vi "LCS kNN.vi"() -> ()   [LabVIEW 2014]
uses:
  <vilib>/Utility/file.llb/Write To Spreadsheet File (string).vi
panel:
  in  "4 groups":string[][](array[string])=[["0 1 0 1 0 3 0", "10", "1"], ["0 -1 1 0 1 0 3 0", "10", "1"], ["0 1 -1 0 1 0 3 0", "10", "1"], ["0 -4 1 0 1 0 3 0", "10", "1"], ["0 1 -4 0 1 0 3 0", "10", "1"], ["0 1 0 -1 1 0 3 0", "10", "1"], ["0 -1 1 0 -1 1 0 3 0", "10", "1"], ["0 1 -1 0 -1 1 0 3 0", "10", "1"], ["0 -4 1 0 -1 1 0 3 0", "10", "1"], ["0 1 -4 0 -1 1 0 3 0", "10", "1"], ["0 1 0 1 -1 0 3 0", "10", "1"], ["0 -1 1 0 1 -1 0 3 0", "10", "1"], ["0 1 -1 0 1 -1 0 3 0", "10", "1"], ["0 -4 1 0 1 -1 0 3 0", "10", "1"], ["0 1 -4 0 1 -1 0 3 0", "10", "1"], ["0 1 0 -4 1 0 3 0", "10", "1"], ["0 -1 1 0 -4 1 0 3 0", "10", "1"], ["0 1 -1 0 -4 1 0 3 0", "10", "1"], ["0 -4 1 0 -4 1 0 3 0", "10", "1"], ["0 1 -4 0 -4 1 0 3 0", "10", "1"], ["0 1 0 1 -4 0 3 0", "10", "1"], ["0 -1 1 0 1 -4 0 3 0", "10", "1"], ["0 1 -1 0 1 -4 0 3 0", "10", "1"], ["0 -4 1 0 1 -4 0 3 0", "10", "1"], ["0 1 -4 0 1 -4 0 3 0", "10", "1"], ["0 1 0 1 0 -2 3 0", "10", "1"], ["0 -1 1 0 1 0 -2 3 0", "10", "1"], ["0 1 -1 0 1 0 -2 3 0", "10", "1"], ["0 -4 1 0 1 0 -2 3 0", "10", "1"], ["0 1 -4 0 1 0 -2 3 0", "10", "1"], ["0 1 0 -1 1 0 -2 3 0", "10", "1"], ["0 -1 1 0 -1 1 0 -2 3 0", "10", "1"], ["0 1 -1 0 -1 1 0 -2 3 0", "10", "1"], ["0 -4 1 0 -1 1 0 -2 3 0", "10", "1"], ["0 1 -4 0 -1 1 0 -2 3 0", "10", "1"], ["0 1 0 1 -1 0 -2 3 0", "10", "1"], ["0 -1 1 0 1 -1 0 -2 3 0", "10", "1"], ["0 1 -1 0 1 -1 0 -2 3 0", "10", "1"], ["0 -4 1 0 1 -1 0 -2 3 0", "10", "1"], ["0 1 -4 0 1 -1 0 -2 3 0", "10", "1"], ["0 1 0 -4 1 0 -2 3 0", "10", "1"], ["0 -1 1 0 -4 1 0 -2 3 0", "10", "1"], ["0 1 -1 0 -4 1 0 -2 3 0", "10", "1"], ["0 -4 1 0 -4 1 0 -2 3 0", "10", "1"], ["0 1 -4 0 -4 1 0 -2 3 0", "10", "1"], ["0 1 0 1 -4 0 -2 3 0", "10", "1"], ["0 -1 1 0 1 -4 0 -2 3 0", "10", "1"], ["0 1 -1 0 1 -4 0 -2 3 0", "10", "1"], ["0 -4 1 0 1 -4 0 -2 3 0", "10", "1"], ["0 1 -4 0 1 -4 0 -2 3 0", "10", "1"], ["0 1 0 1 0 3 -2 0", "10", "1"], ["0 -1 1 0 1 0 3 -2 0", "10", "1"], ["0 1 -1 0 1 0 3 -2 0", "10", "1"], ["0 -4 1 0 1 0 3 -2 0", "10", "1"], ["0 1 -4 0 1 0 3 -2 0", "10", "1"], ["0 1 0 -1 1 0 3 -2 0", "10", "1"], ["0 -1 1 0 -1 1 0 3 -2 0", "10", "1"], ["0 1 -1 0 -1 1 0 3 -2 0", "10", "1"], ["0 -4 1 0 -1 1 0 3 -2 0", "10", "1"], ["0 1 -4 0 -1 1 0 3 -2 0", "10", "1"], ["0 1 0 1 -1 0 3 -2 0", "10", "1"], ["0 -1 1 0 1 -1 0 3 -2 0", "10", "1"], ["0 1 -1 0 1 -1 0 3 -2 0", "10", "1"], ["0 -4 1 0 1 -1 0 3 -2 0", "10", "1"], ["0 1 -4 0 1 -1 0 3 -2 0", "10", "1"], ["0 1 0 -4 1 0 3 -2 0", "10", "1"], ["0 -1 1 0 -4 1 0 3 -2 0", "10", "1"], ["0 1 -1 0 -4 1 0 3 -2 0", "10", "1"], ["0 -4 1 0 -4 1 0 3 -2 0", "10", "1"], ["0 1 -4 0 -4 1 0 3 -2 0", "10", "1"], ["0 1 0 1 -4 0 3 -2 0", "10", "1"], ["0 -1 1 0 1 -4 0 3 -2 0", "10", "1"], ["0 1 -1 0 1 -4 0 3 -2 0", "10", "1"], ["0 -4 1 0 1 -4 0 3 -2 0", "10", "1"], ["0 1 -4 0 1 -4 0 3 -2 0", "10", "1"], ["0 1 0 1 0 -3 3 0", "10", "1"], ["0 -1 1 0 1 0 -3 3 0", "10", "1"], ["0 1 -1 0 1 0 -3 3 0", "10", "1"], ["0 -4 1 0 1 0 -3 3 0", "10", "1"], ["0 1 -4 0 1 0 -3 3 0", "10", "1"], ["0 1 0 -1 1 0 -3 3 0", "10", "1"], ["0 -1 1 0 -1 1 0 -3 3 0", "10", "1"], ["0 1 -1 0 -1 1 0 -3 3 0", "10", "1"], ["0 -4 1 0 -1 1 0 -3 3 0", "10", "1"], ["0 1 -4 0 -1 1 0 -3 3 0", "10", "1"], ["0 1 0 1 -1 0 -3 3 0", "10", "1"], ["0 -1 1 0 1 -1 0 -3 3 0", "10", "1"], ["0 1 -1 0 1 -1 0 -3 3 0", "10", "1"], ["0 -4 1 0 1 -1 0 -3 3 0", "10", "1"], ["0 1 -4 0 1 -1 0 -3 3 0", "10", "1"], ["0 1 0 -4 1 0 -3 3 0", "10", "1"], ["0 -1 1 0 -4 1 0 -3 3 0", "10", "1"], ["0 1 -1 0 -4 1 0 -3 3 0", "10", "1"], ["0 -4 1 0 -4 1 0 -3 3 0", "10", "1"], ["0 1 -4 0 -4 1 0 -3 3 0", "10", "1"], ["0 1 0 1 -4 0 -3 3 0", "10", "1"], ["0 -1 1 0 1 -4 0 -3 3 0", "10", "1"], ["0 1 -1 0 1 -4 0 -3 3 0", "10", "1"], ["0 -4 1 0 1 -4 0 -3 3 0", "10", "1"], ["0 1 -4 0 1 -4 0 -3 3 0", "10", "1"], ["0 1 0 1 0 3 -3 0", "10", "1"], ["0 -1 1 0 1 0 3 -3 0", "10", "1"], ["0 1 -1 0 1 0 3 -3 0", "10", "1"], ["0 -4 1 0 1 0 3 -3 0", "10", "1"], ["0 1 -4 0 1 0 3 -3 0", "10", "1"], ["0 1 0 -1 1 0 3 -3 0", "10", "1"], ["0 -1 1 0 -1 1 0 3 -3 0", "10", "1"], ["0 1 -1 0 -1 1 0 3 -3 0", "10", "1"], ["0 -4 1 0 -1 1 0 3 -3 0", "10", "1"], ["0 1 -4 0 -1 1 0 3 -3 0", "10", "1"], ["0 1 0 1 -1 0 3 -3 0", "10", "1"], ["0 -1 1 0 1 -1 0 3 -3 0", "10", "1"], ["0 1 -1 0 1 -1 0 3 -3 0", "10", "1"], ["0 -4 1 0 1 -1 0 3 -3 0", "10", "1"], ["0 1 -4 0 1 -1 0 3 -3 0", "10", "1"], ["0 1 0 -4 1 0 3 -3 0", "10", "1"], ["0 -1 1 0 -4 1 0 3 -3 0", "10", "1"], ["0 1 -1 0 -4 1 0 3 -3 0", "10", "1"], ["0 -4 1 0 -4 1 0 3 -3 0", "10", "1"], ["0 1 -4 0 -4 1 0 3 -3 0", "10", "1"], ["0 1 0 1 -4 0 3 -3 0", "10", "1"], ["0 -1 1 0 1 -4 0 3 -3 0", "10", "1"], ["0 1 -1 0 1 -4 0 3 -3 0", "10", "1"], ["0 -4 1 0 1 -4 0 3 -3 0", "10", "1"], ["0 1 -4 0 1 -4 0 3 -3 0", "10", "1"], ["0 1 0 3 0 1 0", "10", "2"], ["0 -1 1 0 3 0 1 0", "10", "2"], ["0 1 -1 0 3 0 1 0", "10", "2"], ["0 -4 1 0 3 0 1 0", "10", "2"], ["0 1 -4 0 3 0 1 0", "10", "2"], ["0 1 0 -2 3 0 1 0", "10", "2"], ["0 -1 1 0 -2 3 0 1 0", "10", "2"], ["0 1 -1 0 -2 3 0 1 0", "10", "2"], ["0 -4 1 0 -2 3 0 1 0", "10", "2"], ["0 1 -4 0 -2 3 0 1 0", "10", "2"], ["0 1 0 3 -2 0 1 0", "10", "2"], ["0 -1 1 0 3 -2 0 1 0", "10", "2"], ["0 1 -1 0 3 -2 0 1 0", "10", "2"], ["0 -4 1 0 3 -2 0 1 0", "10", "2"], ["0 1 -4 0 3 -2 0 1 0", "10", "2"], ["0 1 0 -3 3 0 1 0", "10", "2"], ["0 -1 1 0 -3 3 0 1 0", "10", "2"], ["0 1 -1 0 -3 3 0 1 0", "10", "2"], ["0 -4 1 0 -3 3 0 1 0", "10", "2"], ["0 1 -4 0 -3 3 0 1 0", "10", "2"], ["0 1 0 3 -3 0 1 0", "10", "2"], ["0 -1 1 0 3 -3 0 1 0", "10", "2"], ["0 1 -1 0 3 -3 0 1 0", "10", "2"], ["0 -4 1 0 3 -3 0 1 0", "10", "2"], ["0 1 -4 0 3 -3 0 1 0", "10", "2"], ["0 1 0 3 0 -1 1 0", "10", "2"], ["0 -1 1 0 3 0 -1 1 0", "10", "2"], ["0 1 -1 0 3 0 -1 1 0", "10", "2"], ["0 -4 1 0 3 0 -1 1 0", "10", "2"], ["0 1 -4 0 3 0 -1 1 0", "10", "2"], ["0 1 0 -2 3 0 -1 1 0", "10", "2"], ["0 -1 1 0 -2 3 0 -1 1 0", "10", "2"], ["0 1 -1 0 -2 3 0 -1 1 0", "10", "2"], ["0 -4 1 0 -2 3 0 -1 1 0", "10", "2"], ["0 1 -4 0 -2 3 0 -1 1 0", "10", "2"], ["0 1 0 3 -2 0 -1 1 0", "10", "2"], ["0 -1 1 0 3 -2 0 -1 1 0", "10", "2"], ["0 1 -1 0 3 -2 0 -1 1 0", "10", "2"], ["0 -4 1 0 3 -2 0 -1 1 0", "10", "2"], ["0 1 -4 0 3 -2 0 -1 1 0", "10", "2"], ["0 1 0 -3 3 0 -1 1 0", "10", "2"], ["0 -1 1 0 -3 3 0 -1 1 0", "10", "2"], ["0 1 -1 0 -3 3 0 -1 1 0", "10", "2"], ["0 -4 1 0 -3 3 0 -1 1 0", "10", "2"], ["0 1 -4 0 -3 3 0 -1 1 0", "10", "2"], ["0 1 0 3 -3 0 -1 1 0", "10", "2"], ["0 -1 1 0 3 -3 0 -1 1 0", "10", "2"], ["0 1 -1 0 3 -3 0 -1 1 0", "10", "2"], ["0 -4 1 0 3 -3 0 -1 1 0", "10", "2"], ["0 1 -4 0 3 -3 0 -1 1 0", "10", "2"], ["0 1 0 3 0 1 -1 0", "10", "2"], ["0 -1 1 0 3 0 1 -1 0", "10", "2"], ["0 1 -1 0 3 0 1 -1 0", "10", "2"], ["0 -4 1 0 3 0 1 -1 0", "10", "2"], ["0 1 -4 0 3 0 1 -1 0", "10", "2"], ["0 1 0 -2 3 0 1 -1 0", "10", "2"], ["0 -1 1 0 -2 3 0 1 -1 0", "10", "2"], ["0 1 -1 0 -2 3 0 1 -1 0", "10", "2"], ["0 -4 1 0 -2 3 0 1 -1 0", "10", "2"], ["0 1 -4 0 -2 3 0 1 -1 0", "10", "2"], ["0 1 0 3 -2 0 1 -1 0", "10", "2"], ["0 -1 1 0 3 -2 0 1 -1 0", "10", "2"], ["0 1 -1 0 3 -2 0 1 -1 0", "10", "2"], ["0 -4 1 0 3 -2 0 1 -1 0", "10", "2"], ["0 1 -4 0 3 -2 0 1 -1 0", "10", "2"], ["0 1 0 -3 3 0 1 -1 0", "10", "2"], ["0 -1 1 0 -3 3 0 1 -1 0", "10", "2"], ["0 1 -1 0 -3 3 0 1 -1 0", "10", "2"], ["0 -4 1 0 -3 3 0 1 -1 0", "10", "2"], ["0 1 -4 0 -3 3 0 1 -1 0", "10", "2"], ["0 1 0 3 -3 0 1 -1 0", "10", "2"], ["0 -1 1 0 3 -3 0 1 -1 0", "10", "2"], ["0 1 -1 0 3 -3 0 1 -1 0", "10", "2"], ["0 -4 1 0 3 -3 0 1 -1 0", "10", "2"], ["0 1 -4 0 3 -3 0 1 -1 0", "10", "2"], ["0 1 0 3 0 -4 1 0", "10", "2"], ["0 -1 1 0 3 0 -4 1 0", "10", "2"], ["0 1 -1 0 3 0 -4 1 0", "10", "2"], ["0 -4 1 0 3 0 -4 1 0", "10", "2"], ["0 1 -4 0 3 0 -4 1 0", "10", "2"], ["0 1 0 -2 3 0 -4 1 0", "10", "2"], ["0 -1 1 0 -2 3 0 -4 1 0", "10", "2"], ["0 1 -1 0 -2 3 0 -4 1 0", "10", "2"], ["0 -4 1 0 -2 3 0 -4 1 0", "10", "2"], ["0 1 -4 0 -2 3 0 -4 1 0", "10", "2"], ["0 1 0 3 -2 0 -4 1 0", "10", "2"], ["0 -1 1 0 3 -2 0 -4 1 0", "10", "2"], ["0 1 -1 0 3 -2 0 -4 1 0", "10", "2"], ["0 -4 1 0 3 -2 0 -4 1 0", "10", "2"], ["0 1 -4 0 3 -2 0 -4 1 0", "10", "2"], ["0 1 0 -3 3 0 -4 1 0", "10", "2"], ["0 -1 1 0 -3 3 0 -4 1 0", "10", "2"], ["0 1 -1 0 -3 3 0 -4 1 0", "10", "2"], ["0 -4 1 0 -3 3 0 -4 1 0", "10", "2"], ["0 1 -4 0 -3 3 0 -4 1 0", "10", "2"], ["0 1 0 3 -3 0 -4 1 0", "10", "2"], ["0 -1 1 0 3 -3 0 -4 1 0", "10", "2"], ["0 1 -1 0 3 -3 0 -4 1 0", "10", "2"], ["0 -4 1 0 3 -3 0 -4 1 0", "10", "2"], ["0 1 -4 0 3 -3 0 -4 1 0", "10", "2"], ["0 1 0 3 0 1 -4 0", "10", "2"], ["0 -1 1 0 3 0 1 -4 0", "10", "2"], ["0 1 -1 0 3 0 1 -4 0", "10", "2"], ["0 -4 1 0 3 0 1 -4 0", "10", "2"], ["0 1 -4 0 3 0 1 -4 0", "10", "2"], ["0 1 0 -2 3 0 1 -4 0", "10", "2"], ["0 -1 1 0 -2 3 0 1 -4 0", "10", "2"], ["0 1 -1 0 -2 3 0 1 -4 0", "10", "2"], ["0 -4 1 0 -2 3 0 1 -4 0", "10", "2"], ["0 1 -4 0 -2 3 0 1 -4 0", "10", "2"], ["0 1 0 3 -2 0 1 -4 0", "10", "2"], ["0 -1 1 0 3 -2 0 1 -4 0", "10", "2"], ["0 1 -1 0 3 -2 0 1 -4 0", "10", "2"], ["0 -4 1 0 3 -2 0 1 -4 0", "10", "2"], ["0 1 -4 0 3 -2 0 1 -4 0", "10", "2"], ["0 1 0 -3 3 0 1 -4 0", "10", "2"], ["0 -1 1 0 -3 3 0 1 -4 0", "10", "2"], ["0 1 -1 0 -3 3 0 1 -4 0", "10", "2"], ["0 -4 1 0 -3 3 0 1 -4 0", "10", "2"], ["0 1 -4 0 -3 3 0 1 -4 0", "10", "2"], ["0 1 0 3 -3 0 1 -4 0", "10", "2"], ["0 -1 1 0 3 -3 0 1 -4 0", "10", "2"], ["0 1 -1 0 3 -3 0 1 -4 0", "10", "2"], ["0 -4 1 0 3 -3 0 1 -4 0", "10", "2"], ["0 1 -4 0 3 -3 0 1 -4 0", "10", "2"], ["0 3 0 3 0 1 0", "10", "3"], ["0 -2 3 0 3 0 1 0", "10", "3"], ["0 3 -2 0 3 0 1 0", "10", "3"], ["0 -3 3 0 3 0 1 0", "10", "3"], ["0 3-3 0 3 0 1 0", "10", "3"], ["0 3 0 -2 3 0 1 0", "10", "3"], ["0 -2 3 0 -2 3 0 1 0", "10", "3"], ["0 3 -2 0 -2 3 0 1 0", "10", "3"], ["0 -3 3 0 -2 3 0 1 0", "10", "3"], ["0 3-3 0 -2 3 0 1 0", "10", "3"], ["0 3 0 3 -2 0 1 0", "10", "3"], ["0 -2 3 0 3 -2 0 1 0", "10", "3"], ["0 3 -2 0 3 -2 0 1 0", "10", "3"], ["0 -3 3 0 3 -2 0 1 0", "10", "3"], ["0 3-3 0 3 -2 0 1 0", "10", "3"], ["0 3 0 -3 3 0 1 0", "10", "3"], ["0 -2 3 0 -3 3 0 1 0", "10", "3"], ["0 3 -2 0 -3 3 0 1 0", "10", "3"], ["0 -3 3 0 -3 3 0 1 0", "10", "3"], ["0 3-3 0 -3 3 0 1 0", "10", "3"], ["0 3 0 3 -3 0 1 0", "10", "3"], ["0 -2 3 0 3 -3 0 1 0", "10", "3"], ["0 3 -2 0 3 -3 0 1 0", "10", "3"], ["0 -3 3 0 3 -3 0 1 0", "10", "3"], ["0 3-3 0 3 -3 0 1 0", "10", "3"], ["0 3 0 3 0 -1 1 0", "10", "3"], ["0 -2 3 0 3 0 -1 1 0", "10", "3"], ["0 3 -2 0 3 0 -1 1 0", "10", "3"], ["0 -3 3 0 3 0 -1 1 0", "10", "3"], ["0 3-3 0 3 0 -1 1 0", "10", "3"], ["0 3 0 -2 3 0 -1 1 0", "10", "3"], ["0 -2 3 0 -2 3 0 -1 1 0", "10", "3"], ["0 3 -2 0 -2 3 0 -1 1 0", "10", "3"], ["0 -3 3 0 -2 3 0 -1 1 0", "10", "3"], ["0 3-3 0 -2 3 0 -1 1 0", "10", "3"], ["0 3 0 3 -2 0 -1 1 0", "10", "3"], ["0 -2 3 0 3 -2 0 -1 1 0", "10", "3"], ["0 3 -2 0 3 -2 0 -1 1 0", "10", "3"], ["0 -3 3 0 3 -2 0 -1 1 0", "10", "3"], ["0 3-3 0 3 -2 0 -1 1 0", "10", "3"], ["0 3 0 -3 3 0 -1 1 0", "10", "3"], ["0 -2 3 0 -3 3 0 -1 1 0", "10", "3"], ["0 3 -2 0 -3 3 0 -1 1 0", "10", "3"], ["0 -3 3 0 -3 3 0 -1 1 0", "10", "3"], ["0 3-3 0 -3 3 0 -1 1 0", "10", "3"], ["0 3 0 3 -3 0 -1 1 0", "10", "3"], ["0 -2 3 0 3 -3 0 -1 1 0", "10", "3"], ["0 3 -2 0 3 -3 0 -1 1 0", "10", "3"], ["0 -3 3 0 3 -3 0 -1 1 0", "10", "3"], ["0 3-3 0 3 -3 0 -1 1 0", "10", "3"], ["0 3 0 3 0 1 -1 0", "10", "3"], ["0 -2 3 0 3 0 1 -1 0", "10", "3"], ["0 3 -2 0 3 0 1 -1 0", "10", "3"], ["0 -3 3 0 3 0 1 -1 0", "10", "3"], ["0 3-3 0 3 0 1 -1 0", "10", "3"], ["0 3 0 -2 3 0 1 -1 0", "10", "3"], ["0 -2 3 0 -2 3 0 1 -1 0", "10", "3"], ["0 3 -2 0 -2 3 0 1 -1 0", "10", "3"], ["0 -3 3 0 -2 3 0 1 -1 0", "10", "3"], ["0 3-3 0 -2 3 0 1 -1 0", "10", "3"], ["0 3 0 3 -2 0 1 -1 0", "10", "3"], ["0 -2 3 0 3 -2 0 1 -1 0", "10", "3"], ["0 3 -2 0 3 -2 0 1 -1 0", "10", "3"], ["0 -3 3 0 3 -2 0 1 -1 0", "10", "3"], ["0 3-3 0 3 -2 0 1 -1 0", "10", "3"], ["0 3 0 -3 3 0 1 -1 0", "10", "3"], ["0 -2 3 0 -3 3 0 1 -1 0", "10", "3"], ["0 3 -2 0 -3 3 0 1 -1 0", "10", "3"], ["0 -3 3 0 -3 3 0 1 -1 0", "10", "3"], ["0 3-3 0 -3 3 0 1 -1 0", "10", "3"], ["0 3 0 3 -3 0 1 -1 0", "10", "3"], ["0 -2 3 0 3 -3 0 1 -1 0", "10", "3"], ["0 3 -2 0 3 -3 0 1 -1 0", "10", "3"], ["0 -3 3 0 3 -3 0 1 -1 0", "10", "3"], ["0 3-3 0 3 -3 0 1 -1 0", "10", "3"], ["0 3 0 3 0 -4 1 0", "10", "3"], ["0 -2 3 0 3 0 -4 1 0", "10", "3"], ["0 3 -2 0 3 0 -4 1 0", "10", "3"], ["0 -3 3 0 3 0 -4 1 0", "10", "3"], ["0 3-3 0 3 0 -4 1 0", "10", "3"], ["0 3 0 -2 3 0 -4 1 0", "10", "3"], ["0 -2 3 0 -2 3 0 -4 1 0", "10", "3"], ["0 3 -2 0 -2 3 0 -4 1 0", "10", "3"], ["0 -3 3 0 -2 3 0 -4 1 0", "10", "3"], ["0 3-3 0 -2 3 0 -4 1 0", "10", "3"], ["0 3 0 3 -2 0 -4 1 0", "10", "3"], ["0 -2 3 0 3 -2 0 -4 1 0", "10", "3"], ["0 3 -2 0 3 -2 0 -4 1 0", "10", "3"], ["0 -3 3 0 3 -2 0 -4 1 0", "10", "3"], ["0 3-3 0 3 -2 0 -4 1 0", "10", "3"], ["0 3 0 -3 3 0 -4 1 0", "10", "3"], ["0 -2 3 0 -3 3 0 -4 1 0", "10", "3"], ["0 3 -2 0 -3 3 0 -4 1 0", "10", "3"], ["0 -3 3 0 -3 3 0 -4 1 0", "10", "3"], ["0 3-3 0 -3 3 0 -4 1 0", "10", "3"], ["0 3 0 3 -3 0 -4 1 0", "10", "3"], ["0 -2 3 0 3 -3 0 -4 1 0", "10", "3"], ["0 3 -2 0 3 -3 0 -4 1 0", "10", "3"], ["0 -3 3 0 3 -3 0 -4 1 0", "10", "3"], ["0 3-3 0 3 -3 0 -4 1 0", "10", "3"], ["0 3 0 3 0 1 -4 0", "10", "3"], ["0 -2 3 0 3 0 1 -4 0", "10", "3"], ["0 3 -2 0 3 0 1 -4 0", "10", "3"], ["0 -3 3 0 3 0 1 -4 0", "10", "3"], ["0 3-3 0 3 0 1 -4 0", "10", "3"], ["0 3 0 -2 3 0 1 -4 0", "10", "3"], ["0 -2 3 0 -2 3 0 1 -4 0", "10", "3"], ["0 3 -2 0 -2 3 0 1 -4 0", "10", "3"], ["0 -3 3 0 -2 3 0 1 -4 0", "10", "3"], ["0 3-3 0 -2 3 0 1 -4 0", "10", "3"], ["0 3 0 3 -2 0 1 -4 0", "10", "3"], ["0 -2 3 0 3 -2 0 1 -4 0", "10", "3"], ["0 3 -2 0 3 -2 0 1 -4 0", "10", "3"], ["0 -3 3 0 3 -2 0 1 -4 0", "10", "3"], ["0 3-3 0 3 -2 0 1 -4 0", "10", "3"], ["0 3 0 -3 3 0 1 -4 0", "10", "3"], ["0 -2 3 0 -3 3 0 1 -4 0", "10", "3"], ["0 3 -2 0 -3 3 0 1 -4 0", "10", "3"], ["0 -3 3 0 -3 3 0 1 -4 0", "10", "3"], ["0 3-3 0 -3 3 0 1 -4 0", "10", "3"], ["0 3 0 3 -3 0 1 -4 0", "10", "3"], ["0 -2 3 0 3 -3 0 1 -4 0", "10", "3"], ["0 3 -2 0 3 -3 0 1 -4 0", "10", "3"], ["0 -3 3 0 3 -3 0 1 -4 0", "10", "3"], ["0 3-3 0 3 -3 0 1 -4 0", "10", "3"], ["0 3 0 1 0 3 0", "10", "4"], ["0 -2 3 0 1 0 3 0", "10", "4"], ["0 3 -2 0 1 0 3 0", "10", "4"], ["0 -3 3 0 1 0 3 0", "10", "4"], ["0 3-3 0 1 0 3 0", "10", "4"], ["0 3 0 -1 1 0 3 0", "10", "4"], ["0 -2 3 0 -1 1 0 3 0", "10", "4"], ["0 3 -2 0 -1 1 0 3 0", "10", "4"], ["0 -3 3 0 -1 1 0 3 0", "10", "4"], ["0 3-3 0 -1 1 0 3 0", "10", "4"], ["0 3 0 1 -1 0 3 0", "10", "4"], ["0 -2 3 0 1 -1 0 3 0", "10", "4"], ["0 3 -2 0 1 -1 0 3 0", "10", "4"], ["0 -3 3 0 1 -1 0 3 0", "10", "4"], ["0 3-3 0 1 -1 0 3 0", "10", "4"], ["0 3 0 -4 1 0 3 0", "10", "4"], ["0 -2 3 0 -4 1 0 3 0", "10", "4"], ["0 3 -2 0 -4 1 0 3 0", "10", "4"], ["0 -3 3 0 -4 1 0 3 0", "10", "4"], ["0 3-3 0 -4 1 0 3 0", "10", "4"], ["0 3 0 1 -4 0 3 0", "10", "4"], ["0 -2 3 0 1 -4 0 3 0", "10", "4"], ["0 3 -2 0 1 -4 0 3 0", "10", "4"], ["0 -3 3 0 1 -4 0 3 0", "10", "4"], ["0 3-3 0 1 -4 0 3 0", "10", "4"], ["0 3 0 1 0 -2 3 0", "10", "4"], ["0 -2 3 0 1 0 -2 3 0", "10", "4"], ["0 3 -2 0 1 0 -2 3 0", "10", "4"], ["0 -3 3 0 1 0 -2 3 0", "10", "4"], ["0 3-3 0 1 0 -2 3 0", "10", "4"], ["0 3 0 -1 1 0 -2 3 0", "10", "4"], ["0 -2 3 0 -1 1 0 -2 3 0", "10", "4"], ["0 3 -2 0 -1 1 0 -2 3 0", "10", "4"], ["0 -3 3 0 -1 1 0 -2 3 0", "10", "4"], ["0 3-3 0 -1 1 0 -2 3 0", "10", "4"], ["0 3 0 1 -1 0 -2 3 0", "10", "4"], ["0 -2 3 0 1 -1 0 -2 3 0", "10", "4"], ["0 3 -2 0 1 -1 0 -2 3 0", "10", "4"], ["0 -3 3 0 1 -1 0 -2 3 0", "10", "4"], ["0 3-3 0 1 -1 0 -2 3 0", "10", "4"], ["0 3 0 -4 1 0 -2 3 0", "10", "4"], ["0 -2 3 0 -4 1 0 -2 3 0", "10", "4"], ["0 3 -2 0 -4 1 0 -2 3 0", "10", "4"], ["0 -3 3 0 -4 1 0 -2 3 0", "10", "4"], ["0 3-3 0 -4 1 0 -2 3 0", "10", "4"], ["0 3 0 1 -4 0 -2 3 0", "10", "4"], ["0 -2 3 0 1 -4 0 -2 3 0", "10", "4"], ["0 3 -2 0 1 -4 0 -2 3 0", "10", "4"], ["0 -3 3 0 1 -4 0 -2 3 0", "10", "4"], ["0 3-3 0 1 -4 0 -2 3 0", "10", "4"], ["0 3 0 1 0 3 -2 0", "10", "4"], ["0 -2 3 0 1 0 3 -2 0", "10", "4"], ["0 3 -2 0 1 0 3 -2 0", "10", "4"], ["0 -3 3 0 1 0 3 -2 0", "10", "4"], ["0 3-3 0 1 0 3 -2 0", "10", "4"], ["0 3 0 -1 1 0 3 -2 0", "10", "4"], ["0 -2 3 0 -1 1 0 3 -2 0", "10", "4"], ["0 3 -2 0 -1 1 0 3 -2 0", "10", "4"], ["0 -3 3 0 -1 1 0 3 -2 0", "10", "4"], ["0 3-3 0 -1 1 0 3 -2 0", "10", "4"], ["0 3 0 1 -1 0 3 -2 0", "10", "4"], ["0 -2 3 0 1 -1 0 3 -2 0", "10", "4"], ["0 3 -2 0 1 -1 0 3 -2 0", "10", "4"], ["0 -3 3 0 1 -1 0 3 -2 0", "10", "4"], ["0 3-3 0 1 -1 0 3 -2 0", "10", "4"], ["0 3 0 -4 1 0 3 -2 0", "10", "4"], ["0 -2 3 0 -4 1 0 3 -2 0", "10", "4"], ["0 3 -2 0 -4 1 0 3 -2 0", "10", "4"], ["0 -3 3 0 -4 1 0 3 -2 0", "10", "4"], ["0 3-3 0 -4 1 0 3 -2 0", "10", "4"], ["0 3 0 1 -4 0 3 -2 0", "10", "4"], ["0 -2 3 0 1 -4 0 3 -2 0", "10", "4"], ["0 3 -2 0 1 -4 0 3 -2 0", "10", "4"], ["0 -3 3 0 1 -4 0 3 -2 0", "10", "4"], ["0 3-3 0 1 -4 0 3 -2 0", "10", "4"], ["0 3 0 1 0 -3 3 0", "10", "4"], ["0 -2 3 0 1 0 -3 3 0", "10", "4"], ["0 3 -2 0 1 0 -3 3 0", "10", "4"], ["0 -3 3 0 1 0 -3 3 0", "10", "4"], ["0 3-3 0 1 0 -3 3 0", "10", "4"], ["0 3 0 -1 1 0 -3 3 0", "10", "4"], ["0 -2 3 0 -1 1 0 -3 3 0", "10", "4"], ["0 3 -2 0 -1 1 0 -3 3 0", "10", "4"], ["0 -3 3 0 -1 1 0 -3 3 0", "10", "4"], ["0 3-3 0 -1 1 0 -3 3 0", "10", "4"], ["0 3 0 1 -1 0 -3 3 0", "10", "4"], ["0 -2 3 0 1 -1 0 -3 3 0", "10", "4"], ["0 3 -2 0 1 -1 0 -3 3 0", "10", "4"], ["0 -3 3 0 1 -1 0 -3 3 0", "10", "4"], ["0 3-3 0 1 -1 0 -3 3 0", "10", "4"], ["0 3 0 -4 1 0 -3 3 0", "10", "4"], ["0 -2 3 0 -4 1 0 -3 3 0", "10", "4"], ["0 3 -2 0 -4 1 0 -3 3 0", "10", "4"], ["0 -3 3 0 -4 1 0 -3 3 0", "10", "4"], ["0 3-3 0 -4 1 0 -3 3 0", "10", "4"], ["0 3 0 1 -4 0 -3 3 0", "10", "4"], ["0 -2 3 0 1 -4 0 -3 3 0", "10", "4"], ["0 3 -2 0 1 -4 0 -3 3 0", "10", "4"], ["0 -3 3 0 1 -4 0 -3 3 0", "10", "4"], ["0 3-3 0 1 -4 0 -3 3 0", "10", "4"], ["0 3 0 1 0 3 -3 0", "10", "4"], ["0 -2 3 0 1 0 3 -3 0", "10", "4"], ["0 3 -2 0 1 0 3 -3 0", "10", "4"], ["0 -3 3 0 1 0 3 -3 0", "10", "4"], ["0 3-3 0 1 0 3 -3 0", "10", "4"], ["0 3 0 -1 1 0 3 -3 0", "10", "4"], ["0 -2 3 0 -1 1 0 3 -3 0", "10", "4"], ["0 3 -2 0 -1 1 0 3 -3 0", "10", "4"], ["0 -3 3 0 -1 1 0 3 -3 0", "10", "4"], ["0 3-3 0 -1 1 0 3 -3 0", "10", "4"], ["0 3 0 1 -1 0 3 -3 0", "10", "4"], ["0 -2 3 0 1 -1 0 3 -3 0", "10", "4"], ["0 3 -2 0 1 -1 0 3 -3 0", "10", "4"], ["0 -3 3 0 1 -1 0 3 -3 0", "10", "4"], ["0 3-3 0 1 -1 0 3 -3 0", "10", "4"], ["0 3 0 -4 1 0 3 -3 0", "10", "4"], ["0 -2 3 0 -4 1 0 3 -3 0", "10", "4"], ["0 3 -2 0 -4 1 0 3 -3 0", "10", "4"], ["0 -3 3 0 -4 1 0 3 -3 0", "10", "4"], ["0 3-3 0 -4 1 0 3 -3 0", "10", "4"], ["0 3 0 1 -4 0 3 -3 0", "10", "4"], ["0 -2 3 0 1 -4 0 3 -3 0", "10", "4"], ["0 3 -2 0 1 -4 0 3 -3 0", "10", "4"], ["0 -3 3 0 1 -4 0 3 -3 0", "10", "4"], ["0 3-3 0 1 -4 0 3 -3 0", "10", "4"]]
  in  "8 groups":string[][](array[string])=[["0 1 0 1 0 3 0", "10", "1"], ["0 -1 1 0 1 0 3 0", "10", "1"], ["0 1 -1 0 1 0 3 0", "10", "1"], ["0 -4 1 0 1 0 3 0", "10", "1"], ["0 1 -4 0 1 0 3 0", "10", "1"], ["0 1 0 -1 1 0 3 0", "10", "1"], ["0 -1 1 0 -1 1 0 3 0", "10", "1"], ["0 1 -1 0 -1 1 0 3 0", "10", "1"], ["0 -4 1 0 -1 1 0 3 0", "10", "1"], ["0 1 -4 0 -1 1 0 3 0", "10", "1"], ["0 1 0 1 -1 0 3 0", "10", "1"], ["0 -1 1 0 1 -1 0 3 0", "10", "1"], ["0 1 -1 0 1 -1 0 3 0", "10", "1"], ["0 -4 1 0 1 -1 0 3 0", "10", "1"], ["0 1 -4 0 1 -1 0 3 0", "10", "1"], ["0 1 0 -4 1 0 3 0", "10", "1"], ["0 -1 1 0 -4 1 0 3 0", "10", "1"], ["0 1 -1 0 -4 1 0 3 0", "10", "1"], ["0 -4 1 0 -4 1 0 3 0", "10", "1"], ["0 1 -4 0 -4 1 0 3 0", "10", "1"], ["0 1 0 1 -4 0 3 0", "10", "1"], ["0 -1 1 0 1 -4 0 3 0", "10", "1"], ["0 1 -1 0 1 -4 0 3 0", "10", "1"], ["0 -4 1 0 1 -4 0 3 0", "10", "1"], ["0 1 -4 0 1 -4 0 3 0", "10", "1"], ["0 1 0 1 0 -2 3 0", "10", "1"], ["0 -1 1 0 1 0 -2 3 0", "10", "1"], ["0 1 -1 0 1 0 -2 3 0", "10", "1"], ["0 -4 1 0 1 0 -2 3 0", "10", "1"], ["0 1 -4 0 1 0 -2 3 0", "10", "1"], ["0 1 0 -1 1 0 -2 3 0", "10", "1"], ["0 -1 1 0 -1 1 0 -2 3 0", "10", "1"], ["0 1 -1 0 -1 1 0 -2 3 0", "10", "1"], ["0 -4 1 0 -1 1 0 -2 3 0", "10", "1"], ["0 1 -4 0 -1 1 0 -2 3 0", "10", "1"], ["0 1 0 1 -1 0 -2 3 0", "10", "1"], ["0 -1 1 0 1 -1 0 -2 3 0", "10", "1"], ["0 1 -1 0 1 -1 0 -2 3 0", "10", "1"], ["0 -4 1 0 1 -1 0 -2 3 0", "10", "1"], ["0 1 -4 0 1 -1 0 -2 3 0", "10", "1"], ["0 1 0 -4 1 0 -2 3 0", "10", "1"], ["0 -1 1 0 -4 1 0 -2 3 0", "10", "1"], ["0 1 -1 0 -4 1 0 -2 3 0", "10", "1"], ["0 -4 1 0 -4 1 0 -2 3 0", "10", "1"], ["0 1 -4 0 -4 1 0 -2 3 0", "10", "1"], ["0 1 0 1 -4 0 -2 3 0", "10", "1"], ["0 -1 1 0 1 -4 0 -2 3 0", "10", "1"], ["0 1 -1 0 1 -4 0 -2 3 0", "10", "1"], ["0 -4 1 0 1 -4 0 -2 3 0", "10", "1"], ["0 1 -4 0 1 -4 0 -2 3 0", "10", "1"], ["0 1 0 1 0 3 -2 0", "10", "1"], ["0 -1 1 0 1 0 3 -2 0", "10", "1"], ["0 1 -1 0 1 0 3 -2 0", "10", "1"], ["0 -4 1 0 1 0 3 -2 0", "10", "1"], ["0 1 -4 0 1 0 3 -2 0", "10", "1"], ["0 1 0 -1 1 0 3 -2 0", "10", "1"], ["0 -1 1 0 -1 1 0 3 -2 0", "10", "1"], ["0 1 -1 0 -1 1 0 3 -2 0", "10", "1"], ["0 -4 1 0 -1 1 0 3 -2 0", "10", "1"], ["0 1 -4 0 -1 1 0 3 -2 0", "10", "1"], ["0 1 0 1 -1 0 3 -2 0", "10", "1"], ["0 -1 1 0 1 -1 0 3 -2 0", "10", "1"], ["0 1 -1 0 1 -1 0 3 -2 0", "10", "1"], ["0 -4 1 0 1 -1 0 3 -2 0", "10", "1"], ["0 1 -4 0 1 -1 0 3 -2 0", "10", "1"], ["0 1 0 -4 1 0 3 -2 0", "10", "1"], ["0 -1 1 0 -4 1 0 3 -2 0", "10", "1"], ["0 1 -1 0 -4 1 0 3 -2 0", "10", "1"], ["0 -4 1 0 -4 1 0 3 -2 0", "10", "1"], ["0 1 -4 0 -4 1 0 3 -2 0", "10", "1"], ["0 1 0 1 -4 0 3 -2 0", "10", "1"], ["0 -1 1 0 1 -4 0 3 -2 0", "10", "1"], ["0 1 -1 0 1 -4 0 3 -2 0", "10", "1"], ["0 -4 1 0 1 -4 0 3 -2 0", "10", "1"], ["0 1 -4 0 1 -4 0 3 -2 0", "10", "1"], ["0 1 0 1 0 -3 3 0", "10", "1"], ["0 -1 1 0 1 0 -3 3 0", "10", "1"], ["0 1 -1 0 1 0 -3 3 0", "10", "1"], ["0 -4 1 0 1 0 -3 3 0", "10", "1"], ["0 1 -4 0 1 0 -3 3 0", "10", "1"], ["0 1 0 -1 1 0 -3 3 0", "10", "1"], ["0 -1 1 0 -1 1 0 -3 3 0", "10", "1"], ["0 1 -1 0 -1 1 0 -3 3 0", "10", "1"], ["0 -4 1 0 -1 1 0 -3 3 0", "10", "1"], ["0 1 -4 0 -1 1 0 -3 3 0", "10", "1"], ["0 1 0 1 -1 0 -3 3 0", "10", "1"], ["0 -1 1 0 1 -1 0 -3 3 0", "10", "1"], ["0 1 -1 0 1 -1 0 -3 3 0", "10", "1"], ["0 -4 1 0 1 -1 0 -3 3 0", "10", "1"], ["0 1 -4 0 1 -1 0 -3 3 0", "10", "1"], ["0 1 0 -4 1 0 -3 3 0", "10", "1"], ["0 -1 1 0 -4 1 0 -3 3 0", "10", "1"], ["0 1 -1 0 -4 1 0 -3 3 0", "10", "1"], ["0 -4 1 0 -4 1 0 -3 3 0", "10", "1"], ["0 1 -4 0 -4 1 0 -3 3 0", "10", "1"], ["0 1 0 1 -4 0 -3 3 0", "10", "1"], ["0 -1 1 0 1 -4 0 -3 3 0", "10", "1"], ["0 1 -1 0 1 -4 0 -3 3 0", "10", "1"], ["0 -4 1 0 1 -4 0 -3 3 0", "10", "1"], ["0 1 -4 0 1 -4 0 -3 3 0", "10", "1"], ["0 1 0 1 0 3 -3 0", "10", "1"], ["0 -1 1 0 1 0 3 -3 0", "10", "1"], ["0 1 -1 0 1 0 3 -3 0", "10", "1"], ["0 -4 1 0 1 0 3 -3 0", "10", "1"], ["0 1 -4 0 1 0 3 -3 0", "10", "1"], ["0 1 0 -1 1 0 3 -3 0", "10", "1"], ["0 -1 1 0 -1 1 0 3 -3 0", "10", "1"], ["0 1 -1 0 -1 1 0 3 -3 0", "10", "1"], ["0 -4 1 0 -1 1 0 3 -3 0", "10", "1"], ["0 1 -4 0 -1 1 0 3 -3 0", "10", "1"], ["0 1 0 1 -1 0 3 -3 0", "10", "1"], ["0 -1 1 0 1 -1 0 3 -3 0", "10", "1"], ["0 1 -1 0 1 -1 0 3 -3 0", "10", "1"], ["0 -4 1 0 1 -1 0 3 -3 0", "10", "1"], ["0 1 -4 0 1 -1 0 3 -3 0", "10", "1"], ["0 1 0 -4 1 0 3 -3 0", "10", "1"], ["0 -1 1 0 -4 1 0 3 -3 0", "10", "1"], ["0 1 -1 0 -4 1 0 3 -3 0", "10", "1"], ["0 -4 1 0 -4 1 0 3 -3 0", "10", "1"], ["0 1 -4 0 -4 1 0 3 -3 0", "10", "1"], ["0 1 0 1 -4 0 3 -3 0", "10", "1"], ["0 -1 1 0 1 -4 0 3 -3 0", "10", "1"], ["0 1 -1 0 1 -4 0 3 -3 0", "10", "1"], ["0 -4 1 0 1 -4 0 3 -3 0", "10", "1"], ["0 1 -4 0 1 -4 0 3 -3 0", "10", "1"], ["0 1 0 3 0 1 0", "10", "2"], ["0 -1 1 0 3 0 1 0", "10", "2"], ["0 1 -1 0 3 0 1 0", "10", "2"], ["0 -4 1 0 3 0 1 0", "10", "2"], ["0 1 -4 0 3 0 1 0", "10", "2"], ["0 1 0 -2 3 0 1 0", "10", "2"], ["0 -1 1 0 -2 3 0 1 0", "10", "2"], ["0 1 -1 0 -2 3 0 1 0", "10", "2"], ["0 -4 1 0 -2 3 0 1 0", "10", "2"], ["0 1 -4 0 -2 3 0 1 0", "10", "2"], ["0 1 0 3 -2 0 1 0", "10", "2"], ["0 -1 1 0 3 -2 0 1 0", "10", "2"], ["0 1 -1 0 3 -2 0 1 0", "10", "2"], ["0 -4 1 0 3 -2 0 1 0", "10", "2"], ["0 1 -4 0 3 -2 0 1 0", "10", "2"], ["0 1 0 -3 3 0 1 0", "10", "2"], ["0 -1 1 0 -3 3 0 1 0", "10", "2"], ["0 1 -1 0 -3 3 0 1 0", "10", "2"], ["0 -4 1 0 -3 3 0 1 0", "10", "2"], ["0 1 -4 0 -3 3 0 1 0", "10", "2"], ["0 1 0 3 -3 0 1 0", "10", "2"], ["0 -1 1 0 3 -3 0 1 0", "10", "2"], ["0 1 -1 0 3 -3 0 1 0", "10", "2"], ["0 -4 1 0 3 -3 0 1 0", "10", "2"], ["0 1 -4 0 3 -3 0 1 0", "10", "2"], ["0 1 0 3 0 -1 1 0", "10", "2"], ["0 -1 1 0 3 0 -1 1 0", "10", "2"], ["0 1 -1 0 3 0 -1 1 0", "10", "2"], ["0 -4 1 0 3 0 -1 1 0", "10", "2"], ["0 1 -4 0 3 0 -1 1 0", "10", "2"], ["0 1 0 -2 3 0 -1 1 0", "10", "2"], ["0 -1 1 0 -2 3 0 -1 1 0", "10", "2"], ["0 1 -1 0 -2 3 0 -1 1 0", "10", "2"], ["0 -4 1 0 -2 3 0 -1 1 0", "10", "2"], ["0 1 -4 0 -2 3 0 -1 1 0", "10", "2"], ["0 1 0 3 -2 0 -1 1 0", "10", "2"], ["0 -1 1 0 3 -2 0 -1 1 0", "10", "2"], ["0 1 -1 0 3 -2 0 -1 1 0", "10", "2"], ["0 -4 1 0 3 -2 0 -1 1 0", "10", "2"], ["0 1 -4 0 3 -2 0 -1 1 0", "10", "2"], ["0 1 0 -3 3 0 -1 1 0", "10", "2"], ["0 -1 1 0 -3 3 0 -1 1 0", "10", "2"], ["0 1 -1 0 -3 3 0 -1 1 0", "10", "2"], ["0 -4 1 0 -3 3 0 -1 1 0", "10", "2"], ["0 1 -4 0 -3 3 0 -1 1 0", "10", "2"], ["0 1 0 3 -3 0 -1 1 0", "10", "2"], ["0 -1 1 0 3 -3 0 -1 1 0", "10", "2"], ["0 1 -1 0 3 -3 0 -1 1 0", "10", "2"], ["0 -4 1 0 3 -3 0 -1 1 0", "10", "2"], ["0 1 -4 0 3 -3 0 -1 1 0", "10", "2"], ["0 1 0 3 0 1 -1 0", "10", "2"], ["0 -1 1 0 3 0 1 -1 0", "10", "2"], ["0 1 -1 0 3 0 1 -1 0", "10", "2"], ["0 -4 1 0 3 0 1 -1 0", "10", "2"], ["0 1 -4 0 3 0 1 -1 0", "10", "2"], ["0 1 0 -2 3 0 1 -1 0", "10", "2"], ["0 -1 1 0 -2 3 0 1 -1 0", "10", "2"], ["0 1 -1 0 -2 3 0 1 -1 0", "10", "2"], ["0 -4 1 0 -2 3 0 1 -1 0", "10", "2"], ["0 1 -4 0 -2 3 0 1 -1 0", "10", "2"], ["0 1 0 3 -2 0 1 -1 0", "10", "2"], ["0 -1 1 0 3 -2 0 1 -1 0", "10", "2"], ["0 1 -1 0 3 -2 0 1 -1 0", "10", "2"], ["0 -4 1 0 3 -2 0 1 -1 0", "10", "2"], ["0 1 -4 0 3 -2 0 1 -1 0", "10", "2"], ["0 1 0 -3 3 0 1 -1 0", "10", "2"], ["0 -1 1 0 -3 3 0 1 -1 0", "10", "2"], ["0 1 -1 0 -3 3 0 1 -1 0", "10", "2"], ["0 -4 1 0 -3 3 0 1 -1 0", "10", "2"], ["0 1 -4 0 -3 3 0 1 -1 0", "10", "2"], ["0 1 0 3 -3 0 1 -1 0", "10", "2"], ["0 -1 1 0 3 -3 0 1 -1 0", "10", "2"], ["0 1 -1 0 3 -3 0 1 -1 0", "10", "2"], ["0 -4 1 0 3 -3 0 1 -1 0", "10", "2"], ["0 1 -4 0 3 -3 0 1 -1 0", "10", "2"], ["0 1 0 3 0 -4 1 0", "10", "2"], ["0 -1 1 0 3 0 -4 1 0", "10", "2"], ["0 1 -1 0 3 0 -4 1 0", "10", "2"], ["0 -4 1 0 3 0 -4 1 0", "10", "2"], ["0 1 -4 0 3 0 -4 1 0", "10", "2"], ["0 1 0 -2 3 0 -4 1 0", "10", "2"], ["0 -1 1 0 -2 3 0 -4 1 0", "10", "2"], ["0 1 -1 0 -2 3 0 -4 1 0", "10", "2"], ["0 -4 1 0 -2 3 0 -4 1 0", "10", "2"], ["0 1 -4 0 -2 3 0 -4 1 0", "10", "2"], ["0 1 0 3 -2 0 -4 1 0", "10", "2"], ["0 -1 1 0 3 -2 0 -4 1 0", "10", "2"], ["0 1 -1 0 3 -2 0 -4 1 0", "10", "2"], ["0 -4 1 0 3 -2 0 -4 1 0", "10", "2"], ["0 1 -4 0 3 -2 0 -4 1 0", "10", "2"], ["0 1 0 -3 3 0 -4 1 0", "10", "2"], ["0 -1 1 0 -3 3 0 -4 1 0", "10", "2"], ["0 1 -1 0 -3 3 0 -4 1 0", "10", "2"], ["0 -4 1 0 -3 3 0 -4 1 0", "10", "2"], ["0 1 -4 0 -3 3 0 -4 1 0", "10", "2"], ["0 1 0 3 -3 0 -4 1 0", "10", "2"], ["0 -1 1 0 3 -3 0 -4 1 0", "10", "2"], ["0 1 -1 0 3 -3 0 -4 1 0", "10", "2"], ["0 -4 1 0 3 -3 0 -4 1 0", "10", "2"], ["0 1 -4 0 3 -3 0 -4 1 0", "10", "2"], ["0 1 0 3 0 1 -4 0", "10", "2"], ["0 -1 1 0 3 0 1 -4 0", "10", "2"], ["0 1 -1 0 3 0 1 -4 0", "10", "2"], ["0 -4 1 0 3 0 1 -4 0", "10", "2"], ["0 1 -4 0 3 0 1 -4 0", "10", "2"], ["0 1 0 -2 3 0 1 -4 0", "10", "2"], ["0 -1 1 0 -2 3 0 1 -4 0", "10", "2"], ["0 1 -1 0 -2 3 0 1 -4 0", "10", "2"], ["0 -4 1 0 -2 3 0 1 -4 0", "10", "2"], ["0 1 -4 0 -2 3 0 1 -4 0", "10", "2"], ["0 1 0 3 -2 0 1 -4 0", "10", "2"], ["0 -1 1 0 3 -2 0 1 -4 0", "10", "2"], ["0 1 -1 0 3 -2 0 1 -4 0", "10", "2"], ["0 -4 1 0 3 -2 0 1 -4 0", "10", "2"], ["0 1 -4 0 3 -2 0 1 -4 0", "10", "2"], ["0 1 0 -3 3 0 1 -4 0", "10", "2"], ["0 -1 1 0 -3 3 0 1 -4 0", "10", "2"], ["0 1 -1 0 -3 3 0 1 -4 0", "10", "2"], ["0 -4 1 0 -3 3 0 1 -4 0", "10", "2"], ["0 1 -4 0 -3 3 0 1 -4 0", "10", "2"], ["0 1 0 3 -3 0 1 -4 0", "10", "2"], ["0 -1 1 0 3 -3 0 1 -4 0", "10", "2"], ["0 1 -1 0 3 -3 0 1 -4 0", "10", "2"], ["0 -4 1 0 3 -3 0 1 -4 0", "10", "2"], ["0 1 -4 0 3 -3 0 1 -4 0", "10", "2"], ["0 3 0 3 0 1 0", "10", "3"], ["0 -2 3 0 3 0 1 0", "10", "3"], ["0 3 -2 0 3 0 1 0", "10", "3"], ["0 -3 3 0 3 0 1 0", "10", "3"], ["0 3-3 0 3 0 1 0", "10", "3"], ["0 3 0 -2 3 0 1 0", "10", "3"], ["0 -2 3 0 -2 3 0 1 0", "10", "3"], ["0 3 -2 0 -2 3 0 1 0", "10", "3"], ["0 -3 3 0 -2 3 0 1 0", "10", "3"], ["0 3-3 0 -2 3 0 1 0", "10", "3"], ["0 3 0 3 -2 0 1 0", "10", "3"], ["0 -2 3 0 3 -2 0 1 0", "10", "3"], ["0 3 -2 0 3 -2 0 1 0", "10", "3"], ["0 -3 3 0 3 -2 0 1 0", "10", "3"], ["0 3-3 0 3 -2 0 1 0", "10", "3"], ["0 3 0 -3 3 0 1 0", "10", "3"], ["0 -2 3 0 -3 3 0 1 0", "10", "3"], ["0 3 -2 0 -3 3 0 1 0", "10", "3"], ["0 -3 3 0 -3 3 0 1 0", "10", "3"], ["0 3-3 0 -3 3 0 1 0", "10", "3"], ["0 3 0 3 -3 0 1 0", "10", "3"], ["0 -2 3 0 3 -3 0 1 0", "10", "3"], ["0 3 -2 0 3 -3 0 1 0", "10", "3"], ["0 -3 3 0 3 -3 0 1 0", "10", "3"], ["0 3-3 0 3 -3 0 1 0", "10", "3"], ["0 3 0 3 0 -1 1 0", "10", "3"], ["0 -2 3 0 3 0 -1 1 0", "10", "3"], ["0 3 -2 0 3 0 -1 1 0", "10", "3"], ["0 -3 3 0 3 0 -1 1 0", "10", "3"], ["0 3-3 0 3 0 -1 1 0", "10", "3"], ["0 3 0 -2 3 0 -1 1 0", "10", "3"], ["0 -2 3 0 -2 3 0 -1 1 0", "10", "3"], ["0 3 -2 0 -2 3 0 -1 1 0", "10", "3"], ["0 -3 3 0 -2 3 0 -1 1 0", "10", "3"], ["0 3-3 0 -2 3 0 -1 1 0", "10", "3"], ["0 3 0 3 -2 0 -1 1 0", "10", "3"], ["0 -2 3 0 3 -2 0 -1 1 0", "10", "3"], ["0 3 -2 0 3 -2 0 -1 1 0", "10", "3"], ["0 -3 3 0 3 -2 0 -1 1 0", "10", "3"], ["0 3-3 0 3 -2 0 -1 1 0", "10", "3"], ["0 3 0 -3 3 0 -1 1 0", "10", "3"], ["0 -2 3 0 -3 3 0 -1 1 0", "10", "3"], ["0 3 -2 0 -3 3 0 -1 1 0", "10", "3"], ["0 -3 3 0 -3 3 0 -1 1 0", "10", "3"], ["0 3-3 0 -3 3 0 -1 1 0", "10", "3"], ["0 3 0 3 -3 0 -1 1 0", "10", "3"], ["0 -2 3 0 3 -3 0 -1 1 0", "10", "3"], ["0 3 -2 0 3 -3 0 -1 1 0", "10", "3"], ["0 -3 3 0 3 -3 0 -1 1 0", "10", "3"], ["0 3-3 0 3 -3 0 -1 1 0", "10", "3"], ["0 3 0 3 0 1 -1 0", "10", "3"], ["0 -2 3 0 3 0 1 -1 0", "10", "3"], ["0 3 -2 0 3 0 1 -1 0", "10", "3"], ["0 -3 3 0 3 0 1 -1 0", "10", "3"], ["0 3-3 0 3 0 1 -1 0", "10", "3"], ["0 3 0 -2 3 0 1 -1 0", "10", "3"], ["0 -2 3 0 -2 3 0 1 -1 0", "10", "3"], ["0 3 -2 0 -2 3 0 1 -1 0", "10", "3"], ["0 -3 3 0 -2 3 0 1 -1 0", "10", "3"], ["0 3-3 0 -2 3 0 1 -1 0", "10", "3"], ["0 3 0 3 -2 0 1 -1 0", "10", "3"], ["0 -2 3 0 3 -2 0 1 -1 0", "10", "3"], ["0 3 -2 0 3 -2 0 1 -1 0", "10", "3"], ["0 -3 3 0 3 -2 0 1 -1 0", "10", "3"], ["0 3-3 0 3 -2 0 1 -1 0", "10", "3"], ["0 3 0 -3 3 0 1 -1 0", "10", "3"], ["0 -2 3 0 -3 3 0 1 -1 0", "10", "3"], ["0 3 -2 0 -3 3 0 1 -1 0", "10", "3"], ["0 -3 3 0 -3 3 0 1 -1 0", "10", "3"], ["0 3-3 0 -3 3 0 1 -1 0", "10", "3"], ["0 3 0 3 -3 0 1 -1 0", "10", "3"], ["0 -2 3 0 3 -3 0 1 -1 0", "10", "3"], ["0 3 -2 0 3 -3 0 1 -1 0", "10", "3"], ["0 -3 3 0 3 -3 0 1 -1 0", "10", "3"], ["0 3-3 0 3 -3 0 1 -1 0", "10", "3"], ["0 3 0 3 0 -4 1 0", "10", "3"], ["0 -2 3 0 3 0 -4 1 0", "10", "3"], ["0 3 -2 0 3 0 -4 1 0", "10", "3"], ["0 -3 3 0 3 0 -4 1 0", "10", "3"], ["0 3-3 0 3 0 -4 1 0", "10", "3"], ["0 3 0 -2 3 0 -4 1 0", "10", "3"], ["0 -2 3 0 -2 3 0 -4 1 0", "10", "3"], ["0 3 -2 0 -2 3 0 -4 1 0", "10", "3"], ["0 -3 3 0 -2 3 0 -4 1 0", "10", "3"], ["0 3-3 0 -2 3 0 -4 1 0", "10", "3"], ["0 3 0 3 -2 0 -4 1 0", "10", "3"], ["0 -2 3 0 3 -2 0 -4 1 0", "10", "3"], ["0 3 -2 0 3 -2 0 -4 1 0", "10", "3"], ["0 -3 3 0 3 -2 0 -4 1 0", "10", "3"], ["0 3-3 0 3 -2 0 -4 1 0", "10", "3"], ["0 3 0 -3 3 0 -4 1 0", "10", "3"], ["0 -2 3 0 -3 3 0 -4 1 0", "10", "3"], ["0 3 -2 0 -3 3 0 -4 1 0", "10", "3"], ["0 -3 3 0 -3 3 0 -4 1 0", "10", "3"], ["0 3-3 0 -3 3 0 -4 1 0", "10", "3"], ["0 3 0 3 -3 0 -4 1 0", "10", "3"], ["0 -2 3 0 3 -3 0 -4 1 0", "10", "3"], ["0 3 -2 0 3 -3 0 -4 1 0", "10", "3"], ["0 -3 3 0 3 -3 0 -4 1 0", "10", "3"], ["0 3-3 0 3 -3 0 -4 1 0", "10", "3"], ["0 3 0 3 0 1 -4 0", "10", "3"], ["0 -2 3 0 3 0 1 -4 0", "10", "3"], ["0 3 -2 0 3 0 1 -4 0", "10", "3"], ["0 -3 3 0 3 0 1 -4 0", "10", "3"], ["0 3-3 0 3 0 1 -4 0", "10", "3"], ["0 3 0 -2 3 0 1 -4 0", "10", "3"], ["0 -2 3 0 -2 3 0 1 -4 0", "10", "3"], ["0 3 -2 0 -2 3 0 1 -4 0", "10", "3"], ["0 -3 3 0 -2 3 0 1 -4 0", "10", "3"], ["0 3-3 0 -2 3 0 1 -4 0", "10", "3"], ["0 3 0 3 -2 0 1 -4 0", "10", "3"], ["0 -2 3 0 3 -2 0 1 -4 0", "10", "3"], ["0 3 -2 0 3 -2 0 1 -4 0", "10", "3"], ["0 -3 3 0 3 -2 0 1 -4 0", "10", "3"], ["0 3-3 0 3 -2 0 1 -4 0", "10", "3"], ["0 3 0 -3 3 0 1 -4 0", "10", "3"], ["0 -2 3 0 -3 3 0 1 -4 0", "10", "3"], ["0 3 -2 0 -3 3 0 1 -4 0", "10", "3"], ["0 -3 3 0 -3 3 0 1 -4 0", "10", "3"], ["0 3-3 0 -3 3 0 1 -4 0", "10", "3"], ["0 3 0 3 -3 0 1 -4 0", "10", "3"], ["0 -2 3 0 3 -3 0 1 -4 0", "10", "3"], ["0 3 -2 0 3 -3 0 1 -4 0", "10", "3"], ["0 -3 3 0 3 -3 0 1 -4 0", "10", "3"], ["0 3-3 0 3 -3 0 1 -4 0", "10", "3"], ["0 3 0 1 0 3 0", "10", "4"], ["0 -2 3 0 1 0 3 0", "10", "4"], ["0 3 -2 0 1 0 3 0", "10", "4"], ["0 -3 3 0 1 0 3 0", "10", "4"], ["0 3-3 0 1 0 3 0", "10", "4"], ["0 3 0 -1 1 0 3 0", "10", "4"], ["0 -2 3 0 -1 1 0 3 0", "10", "4"], ["0 3 -2 0 -1 1 0 3 0", "10", "4"], ["0 -3 3 0 -1 1 0 3 0", "10", "4"], ["0 3-3 0 -1 1 0 3 0", "10", "4"], ["0 3 0 1 -1 0 3 0", "10", "4"], ["0 -2 3 0 1 -1 0 3 0", "10", "4"], ["0 3 -2 0 1 -1 0 3 0", "10", "4"], ["0 -3 3 0 1 -1 0 3 0", "10", "4"], ["0 3-3 0 1 -1 0 3 0", "10", "4"], ["0 3 0 -4 1 0 3 0", "10", "4"], ["0 -2 3 0 -4 1 0 3 0", "10", "4"], ["0 3 -2 0 -4 1 0 3 0", "10", "4"], ["0 -3 3 0 -4 1 0 3 0", "10", "4"], ["0 3-3 0 -4 1 0 3 0", "10", "4"], ["0 3 0 1 -4 0 3 0", "10", "4"], ["0 -2 3 0 1 -4 0 3 0", "10", "4"], ["0 3 -2 0 1 -4 0 3 0", "10", "4"], ["0 -3 3 0 1 -4 0 3 0", "10", "4"], ["0 3-3 0 1 -4 0 3 0", "10", "4"], ["0 3 0 1 0 -2 3 0", "10", "4"], ["0 -2 3 0 1 0 -2 3 0", "10", "4"], ["0 3 -2 0 1 0 -2 3 0", "10", "4"], ["0 -3 3 0 1 0 -2 3 0", "10", "4"], ["0 3-3 0 1 0 -2 3 0", "10", "4"], ["0 3 0 -1 1 0 -2 3 0", "10", "4"], ["0 -2 3 0 -1 1 0 -2 3 0", "10", "4"], ["0 3 -2 0 -1 1 0 -2 3 0", "10", "4"], ["0 -3 3 0 -1 1 0 -2 3 0", "10", "4"], ["0 3-3 0 -1 1 0 -2 3 0", "10", "4"], ["0 3 0 1 -1 0 -2 3 0", "10", "4"], ["0 -2 3 0 1 -1 0 -2 3 0", "10", "4"], ["0 3 -2 0 1 -1 0 -2 3 0", "10", "4"], ["0 -3 3 0 1 -1 0 -2 3 0", "10", "4"], ["0 3-3 0 1 -1 0 -2 3 0", "10", "4"], ["0 3 0 -4 1 0 -2 3 0", "10", "4"], ["0 -2 3 0 -4 1 0 -2 3 0", "10", "4"], ["0 3 -2 0 -4 1 0 -2 3 0", "10", "4"], ["0 -3 3 0 -4 1 0 -2 3 0", "10", "4"], ["0 3-3 0 -4 1 0 -2 3 0", "10", "4"], ["0 3 0 1 -4 0 -2 3 0", "10", "4"], ["0 -2 3 0 1 -4 0 -2 3 0", "10", "4"], ["0 3 -2 0 1 -4 0 -2 3 0", "10", "4"], ["0 -3 3 0 1 -4 0 -2 3 0", "10", "4"], ["0 3-3 0 1 -4 0 -2 3 0", "10", "4"], ["0 3 0 1 0 3 -2 0", "10", "4"], ["0 -2 3 0 1 0 3 -2 0", "10", "4"], ["0 3 -2 0 1 0 3 -2 0", "10", "4"], ["0 -3 3 0 1 0 3 -2 0", "10", "4"], ["0 3-3 0 1 0 3 -2 0", "10", "4"], ["0 3 0 -1 1 0 3 -2 0", "10", "4"], ["0 -2 3 0 -1 1 0 3 -2 0", "10", "4"], ["0 3 -2 0 -1 1 0 3 -2 0", "10", "4"], ["0 -3 3 0 -1 1 0 3 -2 0", "10", "4"], ["0 3-3 0 -1 1 0 3 -2 0", "10", "4"], ["0 3 0 1 -1 0 3 -2 0", "10", "4"], ["0 -2 3 0 1 -1 0 3 -2 0", "10", "4"], ["0 3 -2 0 1 -1 0 3 -2 0", "10", "4"], ["0 -3 3 0 1 -1 0 3 -2 0", "10", "4"], ["0 3-3 0 1 -1 0 3 -2 0", "10", "4"], ["0 3 0 -4 1 0 3 -2 0", "10", "4"], ["0 -2 3 0 -4 1 0 3 -2 0", "10", "4"], ["0 3 -2 0 -4 1 0 3 -2 0", "10", "4"], ["0 -3 3 0 -4 1 0 3 -2 0", "10", "4"], ["0 3-3 0 -4 1 0 3 -2 0", "10", "4"], ["0 3 0 1 -4 0 3 -2 0", "10", "4"], ["0 -2 3 0 1 -4 0 3 -2 0", "10", "4"], ["0 3 -2 0 1 -4 0 3 -2 0", "10", "4"], ["0 -3 3 0 1 -4 0 3 -2 0", "10", "4"], ["0 3-3 0 1 -4 0 3 -2 0", "10", "4"], ["0 3 0 1 0 -3 3 0", "10", "4"], ["0 -2 3 0 1 0 -3 3 0", "10", "4"], ["0 3 -2 0 1 0 -3 3 0", "10", "4"], ["0 -3 3 0 1 0 -3 3 0", "10", "4"], ["0 3-3 0 1 0 -3 3 0", "10", "4"], ["0 3 0 -1 1 0 -3 3 0", "10", "4"], ["0 -2 3 0 -1 1 0 -3 3 0", "10", "4"], ["0 3 -2 0 -1 1 0 -3 3 0", "10", "4"], ["0 -3 3 0 -1 1 0 -3 3 0", "10", "4"], ["0 3-3 0 -1 1 0 -3 3 0", "10", "4"], ["0 3 0 1 -1 0 -3 3 0", "10", "4"], ["0 -2 3 0 1 -1 0 -3 3 0", "10", "4"], ["0 3 -2 0 1 -1 0 -3 3 0", "10", "4"], ["0 -3 3 0 1 -1 0 -3 3 0", "10", "4"], ["0 3-3 0 1 -1 0 -3 3 0", "10", "4"], ["0 3 0 -4 1 0 -3 3 0", "10", "4"], ["0 -2 3 0 -4 1 0 -3 3 0", "10", "4"], ["0 3 -2 0 -4 1 0 -3 3 0", "10", "4"], ["0 -3 3 0 -4 1 0 -3 3 0", "10", "4"], ["0 3-3 0 -4 1 0 -3 3 0", "10", "4"], ["0 3 0 1 -4 0 -3 3 0", "10", "4"], ["0 -2 3 0 1 -4 0 -3 3 0", "10", "4"], ["0 3 -2 0 1 -4 0 -3 3 0", "10", "4"], ["0 -3 3 0 1 -4 0 -3 3 0", "10", "4"], ["0 3-3 0 1 -4 0 -3 3 0", "10", "4"], ["0 3 0 1 0 3 -3 0", "10", "4"], ["0 -2 3 0 1 0 3 -3 0", "10", "4"], ["0 3 -2 0 1 0 3 -3 0", "10", "4"], ["0 -3 3 0 1 0 3 -3 0", "10", "4"], ["0 3-3 0 1 0 3 -3 0", "10", "4"], ["0 3 0 -1 1 0 3 -3 0", "10", "4"], ["0 -2 3 0 -1 1 0 3 -3 0", "10", "4"], ["0 3 -2 0 -1 1 0 3 -3 0", "10", "4"], ["0 -3 3 0 -1 1 0 3 -3 0", "10", "4"], ["0 3-3 0 -1 1 0 3 -3 0", "10", "4"], ["0 3 0 1 -1 0 3 -3 0", "10", "4"], ["0 -2 3 0 1 -1 0 3 -3 0", "10", "4"], ["0 3 -2 0 1 -1 0 3 -3 0", "10", "4"], ["0 -3 3 0 1 -1 0 3 -3 0", "10", "4"], ["0 3-3 0 1 -1 0 3 -3 0", "10", "4"], ["0 3 0 -4 1 0 3 -3 0", "10", "4"], ["0 -2 3 0 -4 1 0 3 -3 0", "10", "4"], ["0 3 -2 0 -4 1 0 3 -3 0", "10", "4"], ["0 -3 3 0 -4 1 0 3 -3 0", "10", "4"], ["0 3-3 0 -4 1 0 3 -3 0", "10", "4"], ["0 3 0 1 -4 0 3 -3 0", "10", "4"], ["0 -2 3 0 1 -4 0 3 -3 0", "10", "4"], ["0 3 -2 0 1 -4 0 3 -3 0", "10", "4"], ["0 -3 3 0 1 -4 0 3 -3 0", "10", "4"], ["0 3-3 0 1 -4 0 3 -3 0", "10", "4"], ["0 2 0 2 0 4 0", "10", "5"], ["0 -1 2 0 2 0 4 0", "10", "5"], ["0 2 -1 0 2 0 4 0", "10", "5"], ["0 -2 2 0 2 0 4 0", "10", "5"], ["0 2 -2 0 2 0 4 0", "10", "5"], ["0 2 0 -1 2 0 4 0", "10", "5"], ["0 -1 2 0 -1 2 0 4 0", "10", "5"], ["0 2 -1 0 -1 2 0 4 0", "10", "5"], ["0 -2 2 0 -1 2 0 4 0", "10", "5"], ["0 2 -2 0 -1 2 0 4 0", "10", "5"], ["0 2 0 2 -1 0 4 0", "10", "5"], ["0 -1 2 0 2 -1 0 4 0", "10", "5"], ["0 2 -1 0 2 -1 0 4 0", "10", "5"], ["0 -2 2 0 2 -1 0 4 0", "10", "5"], ["0 2 -2 0 2 -1 0 4 0", "10", "5"], ["0 2 0 -2 2 0 4 0", "10", "5"], ["0 -1 2 0 -2 2 0 4 0", "10", "5"], ["0 2 -1 0 -2 2 0 4 0", "10", "5"], ["0 -2 2 0 -2 2 0 4 0", "10", "5"], ["0 2 -2 0 -2 2 0 4 0", "10", "5"], ["0 2 0 2 -2 0 4 0", "10", "5"], ["0 -1 2 0 2 -2 0 4 0", "10", "5"], ["0 2 -1 0 2 -2 0 4 0", "10", "5"], ["0 -2 2 0 2 -2 0 4 0", "10", "5"], ["0 2 -2 0 2 -2 0 4 0", "10", "5"], ["0 2 0 2 0 -3 4 0", "10", "5"], ["0 -1 2 0 2 0 -3 4 0", "10", "5"], ["0 2 -1 0 2 0 -3 4 0", "10", "5"], ["0 -2 2 0 2 0 -3 4 0", "10", "5"], ["0 2 -2 0 2 0 -3 4 0", "10", "5"], ["0 2 0 -1 2 0 -3 4 0", "10", "5"], ["0 -1 2 0 -1 2 0 -3 4 0", "10", "5"], ["0 2 -1 0 -1 2 0 -3 4 0", "10", "5"], ["0 -2 2 0 -1 2 0 -3 4 0", "10", "5"], ["0 2 -2 0 -1 2 0 -3 4 0", "10", "5"], ["0 2 0 2 -1 0 -3 4 0", "10", "5"], ["0 -1 2 0 2 -1 0 -3 4 0", "10", "5"], ["0 2 -1 0 2 -1 0 -3 4 0", "10", "5"], ["0 -2 2 0 2 -1 0 -3 4 0", "10", "5"], ["0 2 -2 0 2 -1 0 -3 4 0", "10", "5"], ["0 2 0 -2 2 0 -3 4 0", "10", "5"], ["0 -1 2 0 -2 2 0 -3 4 0", "10", "5"], ["0 2 -1 0 -2 2 0 -3 4 0", "10", "5"], ["0 -2 2 0 -2 2 0 -3 4 0", "10", "5"], ["0 2 -2 0 -2 2 0 -3 4 0", "10", "5"], ["0 2 0 2 -2 0 -3 4 0", "10", "5"], ["0 -1 2 0 2 -2 0 -3 4 0", "10", "5"], ["0 2 -1 0 2 -2 0 -3 4 0", "10", "5"], ["0 -2 2 0 2 -2 0 -3 4 0", "10", "5"], ["0 2 -2 0 2 -2 0 -3 4 0", "10", "5"], ["0 2 0 2 0 4 -3 0", "10", "5"], ["0 -1 2 0 2 0 4 -3 0", "10", "5"], ["0 2 -1 0 2 0 4 -3 0", "10", "5"], ["0 -2 2 0 2 0 4 -3 0", "10", "5"], ["0 2 -2 0 2 0 4 -3 0", "10", "5"], ["0 2 0 -1 2 0 4 -3 0", "10", "5"], ["0 -1 2 0 -1 2 0 4 -3 0", "10", "5"], ["0 2 -1 0 -1 2 0 4 -3 0", "10", "5"], ["0 -2 2 0 -1 2 0 4 -3 0", "10", "5"], ["0 2 -2 0 -1 2 0 4 -3 0", "10", "5"], ["0 2 0 2 -1 0 4 -3 0", "10", "5"], ["0 -1 2 0 2 -1 0 4 -3 0", "10", "5"], ["0 2 -1 0 2 -1 0 4 -3 0", "10", "5"], ["0 -2 2 0 2 -1 0 4 -3 0", "10", "5"], ["0 2 -2 0 2 -1 0 4 -3 0", "10", "5"], ["0 2 0 -2 2 0 4 -3 0", "10", "5"], ["0 -1 2 0 -2 2 0 4 -3 0", "10", "5"], ["0 2 -1 0 -2 2 0 4 -3 0", "10", "5"], ["0 -2 2 0 -2 2 0 4 -3 0", "10", "5"], ["0 2 -2 0 -2 2 0 4 -3 0", "10", "5"], ["0 2 0 2 -2 0 4 -3 0", "10", "5"], ["0 -1 2 0 2 -2 0 4 -3 0", "10", "5"], ["0 2 -1 0 2 -2 0 4 -3 0", "10", "5"], ["0 -2 2 0 2 -2 0 4 -3 0", "10", "5"], ["0 2 -2 0 2 -2 0 4 -3 0", "10", "5"], ["0 2 0 2 0 -4 4 0", "10", "5"], ["0 -1 2 0 2 0 -4 4 0", "10", "5"], ["0 2 -1 0 2 0 -4 4 0", "10", "5"], ["0 -2 2 0 2 0 -4 4 0", "10", "5"], ["0 2 -2 0 2 0 -4 4 0", "10", "5"], ["0 2 0 -1 2 0 -4 4 0", "10", "5"], ["0 -1 2 0 -1 2 0 -4 4 0", "10", "5"], ["0 2 -1 0 -1 2 0 -4 4 0", "10", "5"], ["0 -2 2 0 -1 2 0 -4 4 0", "10", "5"], ["0 2 -2 0 -1 2 0 -4 4 0", "10", "5"], ["0 2 0 2 -1 0 -4 4 0", "10", "5"], ["0 -1 2 0 2 -1 0 -4 4 0", "10", "5"], ["0 2 -1 0 2 -1 0 -4 4 0", "10", "5"], ["0 -2 2 0 2 -1 0 -4 4 0", "10", "5"], ["0 2 -2 0 2 -1 0 -4 4 0", "10", "5"], ["0 2 0 -2 2 0 -4 4 0", "10", "5"], ["0 -1 2 0 -2 2 0 -4 4 0", "10", "5"], ["0 2 -1 0 -2 2 0 -4 4 0", "10", "5"], ["0 -2 2 0 -2 2 0 -4 4 0", "10", "5"], ["0 2 -2 0 -2 2 0 -4 4 0", "10", "5"], ["0 2 0 2 -2 0 -4 4 0", "10", "5"], ["0 -1 2 0 2 -2 0 -4 4 0", "10", "5"], ["0 2 -1 0 2 -2 0 -4 4 0", "10", "5"], ["0 -2 2 0 2 -2 0 -4 4 0", "10", "5"], ["0 2 -2 0 2 -2 0 -4 4 0", "10", "5"], ["0 2 0 2 0 4 -4 0", "10", "5"], ["0 -1 2 0 2 0 4 -4 0", "10", "5"], ["0 2 -1 0 2 0 4 -4 0", "10", "5"], ["0 -2 2 0 2 0 4 -4 0", "10", "5"], ["0 2 -2 0 2 0 4 -4 0", "10", "5"], ["0 2 0 -1 2 0 4 -4 0", "10", "5"], ["0 -1 2 0 -1 2 0 4 -4 0", "10", "5"], ["0 2 -1 0 -1 2 0 4 -4 0", "10", "5"], ["0 -2 2 0 -1 2 0 4 -4 0", "10", "5"], ["0 2 -2 0 -1 2 0 4 -4 0", "10", "5"], ["0 2 0 2 -1 0 4 -4 0", "10", "5"], ["0 -1 2 0 2 -1 0 4 -4 0", "10", "5"], ["0 2 -1 0 2 -1 0 4 -4 0", "10", "5"], ["0 -2 2 0 2 -1 0 4 -4 0", "10", "5"], ["0 2 -2 0 2 -1 0 4 -4 0", "10", "5"], ["0 2 0 -2 2 0 4 -4 0", "10", "5"], ["0 -1 2 0 -2 2 0 4 -4 0", "10", "5"], ["0 2 -1 0 -2 2 0 4 -4 0", "10", "5"], ["0 -2 2 0 -2 2 0 4 -4 0", "10", "5"], ["0 2 -2 0 -2 2 0 4 -4 0", "10", "5"], ["0 2 0 2 -2 0 4 -4 0", "10", "5"], ["0 -1 2 0 2 -2 0 4 -4 0", "10", "5"], ["0 2 -1 0 2 -2 0 4 -4 0", "10", "5"], ["0 -2 2 0 2 -2 0 4 -4 0", "10", "5"], ["0 2 -2 0 2 -2 0 4 -4 0", "10", "5"], ["0 2 0 4 0 2 0", "10", "6"], ["0 -1 2 0 4 0 2 0", "10", "6"], ["0 2 -1 0 4 0 2 0", "10", "6"], ["0 -2 2 0 4 0 2 0", "10", "6"], ["0 2 -2 0 4 0 2 0", "10", "6"], ["0 2 0 -3 4 0 2 0", "10", "6"], ["0 -1 2 0 -3 4 0 2 0", "10", "6"], ["0 2 -1 0 -3 4 0 2 0", "10", "6"], ["0 -2 2 0 -3 4 0 2 0", "10", "6"], ["0 2 -2 0 -3 4 0 2 0", "10", "6"], ["0 2 0 4 -3 0 2 0", "10", "6"], ["0 -1 2 0 4 -3 0 2 0", "10", "6"], ["0 2 -1 0 4 -3 0 2 0", "10", "6"], ["0 -2 2 0 4 -3 0 2 0", "10", "6"], ["0 2 -2 0 4 -3 0 2 0", "10", "6"], ["0 2 0 -4 4 0 2 0", "10", "6"], ["0 -1 2 0 -4 4 0 2 0", "10", "6"], ["0 2 -1 0 -4 4 0 2 0", "10", "6"], ["0 -2 2 0 -4 4 0 2 0", "10", "6"], ["0 2 -2 0 -4 4 0 2 0", "10", "6"], ["0 2 0 4 -4 0 2 0", "10", "6"], ["0 -1 2 0 4 -4 0 2 0", "10", "6"], ["0 2 -1 0 4 -4 0 2 0", "10", "6"], ["0 -2 2 0 4 -4 0 2 0", "10", "6"], ["0 2 -2 0 4 -4 0 2 0", "10", "6"], ["0 2 0 4 0 -1 2 0", "10", "6"], ["0 -1 2 0 4 0 -1 2 0", "10", "6"], ["0 2 -1 0 4 0 -1 2 0", "10", "6"], ["0 -2 2 0 4 0 -1 2 0", "10", "6"], ["0 2 -2 0 4 0 -1 2 0", "10", "6"], ["0 2 0 -3 4 0 -1 2 0", "10", "6"], ["0 -1 2 0 -3 4 0 -1 2 0", "10", "6"], ["0 2 -1 0 -3 4 0 -1 2 0", "10", "6"], ["0 -2 2 0 -3 4 0 -1 2 0", "10", "6"], ["0 2 -2 0 -3 4 0 -1 2 0", "10", "6"], ["0 2 0 4 -3 0 -1 2 0", "10", "6"], ["0 -1 2 0 4 -3 0 -1 2 0", "10", "6"], ["0 2 -1 0 4 -3 0 -1 2 0", "10", "6"], ["0 -2 2 0 4 -3 0 -1 2 0", "10", "6"], ["0 2 -2 0 4 -3 0 -1 2 0", "10", "6"], ["0 2 0 -4 4 0 -1 2 0", "10", "6"], ["0 -1 2 0 -4 4 0 -1 2 0", "10", "6"], ["0 2 -1 0 -4 4 0 -1 2 0", "10", "6"], ["0 -2 2 0 -4 4 0 -1 2 0", "10", "6"], ["0 2 -2 0 -4 4 0 -1 2 0", "10", "6"], ["0 2 0 4 -4 0 -1 2 0", "10", "6"], ["0 -1 2 0 4 -4 0 -1 2 0", "10", "6"], ["0 2 -1 0 4 -4 0 -1 2 0", "10", "6"], ["0 -2 2 0 4 -4 0 -1 2 0", "10", "6"], ["0 2 -2 0 4 -4 0 -1 2 0", "10", "6"], ["0 2 0 4 0 2 -1 0", "10", "6"], ["0 -1 2 0 4 0 2 -1 0", "10", "6"], ["0 2 -1 0 4 0 2 -1 0", "10", "6"], ["0 -2 2 0 4 0 2 -1 0", "10", "6"], ["0 2 -2 0 4 0 2 -1 0", "10", "6"], ["0 2 0 -3 4 0 2 -1 0", "10", "6"], ["0 -1 2 0 -3 4 0 2 -1 0", "10", "6"], ["0 2 -1 0 -3 4 0 2 -1 0", "10", "6"], ["0 -2 2 0 -3 4 0 2 -1 0", "10", "6"], ["0 2 -2 0 -3 4 0 2 -1 0", "10", "6"], ["0 2 0 4 -3 0 2 -1 0", "10", "6"], ["0 -1 2 0 4 -3 0 2 -1 0", "10", "6"], ["0 2 -1 0 4 -3 0 2 -1 0", "10", "6"], ["0 -2 2 0 4 -3 0 2 -1 0", "10", "6"], ["0 2 -2 0 4 -3 0 2 -1 0", "10", "6"], ["0 2 0 -4 4 0 2 -1 0", "10", "6"], ["0 -1 2 0 -4 4 0 2 -1 0", "10", "6"], ["0 2 -1 0 -4 4 0 2 -1 0", "10", "6"], ["0 -2 2 0 -4 4 0 2 -1 0", "10", "6"], ["0 2 -2 0 -4 4 0 2 -1 0", "10", "6"], ["0 2 0 4 -4 0 2 -1 0", "10", "6"], ["0 -1 2 0 4 -4 0 2 -1 0", "10", "6"], ["0 2 -1 0 4 -4 0 2 -1 0", "10", "6"], ["0 -2 2 0 4 -4 0 2 -1 0", "10", "6"], ["0 2 -2 0 4 -4 0 2 -1 0", "10", "6"], ["0 2 0 4 0 -2 2 0", "10", "6"], ["0 -1 2 0 4 0 -2 2 0", "10", "6"], ["0 2 -1 0 4 0 -2 2 0", "10", "6"], ["0 -2 2 0 4 0 -2 2 0", "10", "6"], ["0 2 -2 0 4 0 -2 2 0", "10", "6"], ["0 2 0 -3 4 0 -2 2 0", "10", "6"], ["0 -1 2 0 -3 4 0 -2 2 0", "10", "6"], ["0 2 -1 0 -3 4 0 -2 2 0", "10", "6"], ["0 -2 2 0 -3 4 0 -2 2 0", "10", "6"], ["0 2 -2 0 -3 4 0 -2 2 0", "10", "6"], ["0 2 0 4 -3 0 -2 2 0", "10", "6"], ["0 -1 2 0 4 -3 0 -2 2 0", "10", "6"], ["0 2 -1 0 4 -3 0 -2 2 0", "10", "6"], ["0 -2 2 0 4 -3 0 -2 2 0", "10", "6"], ["0 2 -2 0 4 -3 0 -2 2 0", "10", "6"], ["0 2 0 -4 4 0 -2 2 0", "10", "6"], ["0 -1 2 0 -4 4 0 -2 2 0", "10", "6"], ["0 2 -1 0 -4 4 0 -2 2 0", "10", "6"], ["0 -2 2 0 -4 4 0 -2 2 0", "10", "6"], ["0 2 -2 0 -4 4 0 -2 2 0", "10", "6"], ["0 2 0 4 -4 0 -2 2 0", "10", "6"], ["0 -1 2 0 4 -4 0 -2 2 0", "10", "6"], ["0 2 -1 0 4 -4 0 -2 2 0", "10", "6"], ["0 -2 2 0 4 -4 0 -2 2 0", "10", "6"], ["0 2 -2 0 4 -4 0 -2 2 0", "10", "6"], ["0 2 0 4 0 2 -2 0", "10", "6"], ["0 -1 2 0 4 0 2 -2 0", "10", "6"], ["0 2 -1 0 4 0 2 -2 0", "10", "6"], ["0 -2 2 0 4 0 2 -2 0", "10", "6"], ["0 2 -2 0 4 0 2 -2 0", "10", "6"], ["0 2 0 -3 4 0 2 -2 0", "10", "6"], ["0 -1 2 0 -3 4 0 2 -2 0", "10", "6"], ["0 2 -1 0 -3 4 0 2 -2 0", "10", "6"], ["0 -2 2 0 -3 4 0 2 -2 0", "10", "6"], ["0 2 -2 0 -3 4 0 2 -2 0", "10", "6"], ["0 2 0 4 -3 0 2 -2 0", "10", "6"], ["0 -1 2 0 4 -3 0 2 -2 0", "10", "6"], ["0 2 -1 0 4 -3 0 2 -2 0", "10", "6"], ["0 -2 2 0 4 -3 0 2 -2 0", "10", "6"], ["0 2 -2 0 4 -3 0 2 -2 0", "10", "6"], ["0 2 0 -4 4 0 2 -2 0", "10", "6"], ["0 -1 2 0 -4 4 0 2 -2 0", "10", "6"], ["0 2 -1 0 -4 4 0 2 -2 0", "10", "6"], ["0 -2 2 0 -4 4 0 2 -2 0", "10", "6"], ["0 2 -2 0 -4 4 0 2 -2 0", "10", "6"], ["0 2 0 4 -4 0 2 -2 0", "10", "6"], ["0 -1 2 0 4 -4 0 2 -2 0", "10", "6"], ["0 2 -1 0 4 -4 0 2 -2 0", "10", "6"], ["0 -2 2 0 4 -4 0 2 -2 0", "10", "6"], ["0 2 -2 0 4 -4 0 2 -2 0", "10", "6"], ["0 4 0 4 0 2 0", "10", "7"], ["0 -3 4 0 4 0 2 0", "10", "7"], ["0 4 -3 0 4 0 2 0", "10", "7"], ["0 -4 4 0 4 0 2 0", "10", "7"], ["0 4 -4 0 4 0 2 0", "10", "7"], ["0 4 0 -3 4 0 2 0", "10", "7"], ["0 -3 4 0 -3 4 0 2 0", "10", "7"], ["0 4 -3 0 -3 4 0 2 0", "10", "7"], ["0 -4 4 0 -3 4 0 2 0", "10", "7"], ["0 4 -4 0 -3 4 0 2 0", "10", "7"], ["0 4 0 4 -3 0 2 0", "10", "7"], ["0 -3 4 0 4 -3 0 2 0", "10", "7"], ["0 4 -3 0 4 -3 0 2 0", "10", "7"], ["0 -4 4 0 4 -3 0 2 0", "10", "7"], ["0 4 -4 0 4 -3 0 2 0", "10", "7"], ["0 4 0 -4 4 0 2 0", "10", "7"], ["0 -3 4 0 -4 4 0 2 0", "10", "7"], ["0 4 -3 0 -4 4 0 2 0", "10", "7"], ["0 -4 4 0 -4 4 0 2 0", "10", "7"], ["0 4 -4 0 -4 4 0 2 0", "10", "7"], ["0 4 0 4 -4 0 2 0", "10", "7"], ["0 -3 4 0 4 -4 0 2 0", "10", "7"], ["0 4 -3 0 4 -4 0 2 0", "10", "7"], ["0 -4 4 0 4 -4 0 2 0", "10", "7"], ["0 4 -4 0 4 -4 0 2 0", "10", "7"], ["0 4 0 4 0 -1 2 0", "10", "7"], ["0 -3 4 0 4 0 -1 2 0", "10", "7"], ["0 4 -3 0 4 0 -1 2 0", "10", "7"], ["0 -4 4 0 4 0 -1 2 0", "10", "7"], ["0 4 -4 0 4 0 -1 2 0", "10", "7"], ["0 4 0 -3 4 0 -1 2 0", "10", "7"], ["0 -3 4 0 -3 4 0 -1 2 0", "10", "7"], ["0 4 -3 0 -3 4 0 -1 2 0", "10", "7"], ["0 -4 4 0 -3 4 0 -1 2 0", "10", "7"], ["0 4 -4 0 -3 4 0 -1 2 0", "10", "7"], ["0 4 0 4 -3 0 -1 2 0", "10", "7"], ["0 -3 4 0 4 -3 0 -1 2 0", "10", "7"], ["0 4 -3 0 4 -3 0 -1 2 0", "10", "7"], ["0 -4 4 0 4 -3 0 -1 2 0", "10", "7"], ["0 4 -4 0 4 -3 0 -1 2 0", "10", "7"], ["0 4 0 -4 4 0 -1 2 0", "10", "7"], ["0 -3 4 0 -4 4 0 -1 2 0", "10", "7"], ["0 4 -3 0 -4 4 0 -1 2 0", "10", "7"], ["0 -4 4 0 -4 4 0 -1 2 0", "10", "7"], ["0 4 -4 0 -4 4 0 -1 2 0", "10", "7"], ["0 4 0 4 -4 0 -1 2 0", "10", "7"], ["0 -3 4 0 4 -4 0 -1 2 0", "10", "7"], ["0 4 -3 0 4 -4 0 -1 2 0", "10", "7"], ["0 -4 4 0 4 -4 0 -1 2 0", "10", "7"], ["0 4 -4 0 4 -4 0 -1 2 0", "10", "7"], ["0 4 0 4 0 2 -1 0", "10", "7"], ["0 -3 4 0 4 0 2 -1 0", "10", "7"], ["0 4 -3 0 4 0 2 -1 0", "10", "7"], ["0 -4 4 0 4 0 2 -1 0", "10", "7"], ["0 4 -4 0 4 0 2 -1 0", "10", "7"], ["0 4 0 -3 4 0 2 -1 0", "10", "7"], ["0 -3 4 0 -3 4 0 2 -1 0", "10", "7"], ["0 4 -3 0 -3 4 0 2 -1 0", "10", "7"], ["0 -4 4 0 -3 4 0 2 -1 0", "10", "7"], ["0 4 -4 0 -3 4 0 2 -1 0", "10", "7"], ["0 4 0 4 -3 0 2 -1 0", "10", "7"], ["0 -3 4 0 4 -3 0 2 -1 0", "10", "7"], ["0 4 -3 0 4 -3 0 2 -1 0", "10", "7"], ["0 -4 4 0 4 -3 0 2 -1 0", "10", "7"], ["0 4 -4 0 4 -3 0 2 -1 0", "10", "7"], ["0 4 0 -4 4 0 2 -1 0", "10", "7"], ["0 -3 4 0 -4 4 0 2 -1 0", "10", "7"], ["0 4 -3 0 -4 4 0 2 -1 0", "10", "7"], ["0 -4 4 0 -4 4 0 2 -1 0", "10", "7"], ["0 4 -4 0 -4 4 0 2 -1 0", "10", "7"], ["0 4 0 4 -4 0 2 -1 0", "10", "7"], ["0 -3 4 0 4 -4 0 2 -1 0", "10", "7"], ["0 4 -3 0 4 -4 0 2 -1 0", "10", "7"], ["0 -4 4 0 4 -4 0 2 -1 0", "10", "7"], ["0 4 -4 0 4 -4 0 2 -1 0", "10", "7"], ["0 4 0 4 0 -2 2 0", "10", "7"], ["0 -3 4 0 4 0 -2 2 0", "10", "7"], ["0 4 -3 0 4 0 -2 2 0", "10", "7"], ["0 -4 4 0 4 0 -2 2 0", "10", "7"], ["0 4 -4 0 4 0 -2 2 0", "10", "7"], ["0 4 0 -3 4 0 -2 2 0", "10", "7"], ["0 -3 4 0 -3 4 0 -2 2 0", "10", "7"], ["0 4 -3 0 -3 4 0 -2 2 0", "10", "7"], ["0 -4 4 0 -3 4 0 -2 2 0", "10", "7"], ["0 4 -4 0 -3 4 0 -2 2 0", "10", "7"], ["0 4 0 4 -3 0 -2 2 0", "10", "7"], ["0 -3 4 0 4 -3 0 -2 2 0", "10", "7"], ["0 4 -3 0 4 -3 0 -2 2 0", "10", "7"], ["0 -4 4 0 4 -3 0 -2 2 0", "10", "7"], ["0 4 -4 0 4 -3 0 -2 2 0", "10", "7"], ["0 4 0 -4 4 0 -2 2 0", "10", "7"], ["0 -3 4 0 -4 4 0 -2 2 0", "10", "7"], ["0 4 -3 0 -4 4 0 -2 2 0", "10", "7"], ["0 -4 4 0 -4 4 0 -2 2 0", "10", "7"], ["0 4 -4 0 -4 4 0 -2 2 0", "10", "7"], ["0 4 0 4 -4 0 -2 2 0", "10", "7"], ["0 -3 4 0 4 -4 0 -2 2 0", "10", "7"], ["0 4 -3 0 4 -4 0 -2 2 0", "10", "7"], ["0 -4 4 0 4 -4 0 -2 2 0", "10", "7"], ["0 4 -4 0 4 -4 0 -2 2 0", "10", "7"], ["0 4 0 4 0 2 -2 0", "10", "7"], ["0 -3 4 0 4 0 2 -2 0", "10", "7"], ["0 4 -3 0 4 0 2 -2 0", "10", "7"], ["0 -4 4 0 4 0 2 -2 0", "10", "7"], ["0 4 -4 0 4 0 2 -2 0", "10", "7"], ["0 4 0 -3 4 0 2 -2 0", "10", "7"], ["0 -3 4 0 -3 4 0 2 -2 0", "10", "7"], ["0 4 -3 0 -3 4 0 2 -2 0", "10", "7"], ["0 -4 4 0 -3 4 0 2 -2 0", "10", "7"], ["0 4 -4 0 -3 4 0 2 -2 0", "10", "7"], ["0 4 0 4 -3 0 2 -2 0", "10", "7"], ["0 -3 4 0 4 -3 0 2 -2 0", "10", "7"], ["0 4 -3 0 4 -3 0 2 -2 0", "10", "7"], ["0 -4 4 0 4 -3 0 2 -2 0", "10", "7"], ["0 4 -4 0 4 -3 0 2 -2 0", "10", "7"], ["0 4 0 -4 4 0 2 -2 0", "10", "7"], ["0 -3 4 0 -4 4 0 2 -2 0", "10", "7"], ["0 4 -3 0 -4 4 0 2 -2 0", "10", "7"], ["0 -4 4 0 -4 4 0 2 -2 0", "10", "7"], ["0 4 -4 0 -4 4 0 2 -2 0", "10", "7"], ["0 4 0 4 -4 0 2 -2 0", "10", "7"], ["0 -3 4 0 4 -4 0 2 -2 0", "10", "7"], ["0 4 -3 0 4 -4 0 2 -2 0", "10", "7"], ["0 -4 4 0 4 -4 0 2 -2 0", "10", "7"], ["0 4 -4 0 4 -4 0 2 -2 0", "10", "7"], ["0 4 0 2 0 4 0", "10", "8"], ["0 -3 4 0 2 0 4 0", "10", "8"], ["0 4 -3 0 2 0 4 0", "10", "8"], ["0 -4 4 0 2 0 4 0", "10", "8"], ["0 4 -4 0 2 0 4 0", "10", "8"], ["0 4 0 -1 2 0 4 0", "10", "8"], ["0 -3 4 0 -1 2 0 4 0", "10", "8"], ["0 4 -3 0 -1 2 0 4 0", "10", "8"], ["0 -4 4 0 -1 2 0 4 0", "10", "8"], ["0 4 -4 0 -1 2 0 4 0", "10", "8"], ["0 4 0 2 -1 0 4 0", "10", "8"], ["0 -3 4 0 2 -1 0 4 0", "10", "8"], ["0 4 -3 0 2 -1 0 4 0", "10", "8"], ["0 -4 4 0 2 -1 0 4 0", "10", "8"], ["0 4 -4 0 2 -1 0 4 0", "10", "8"], ["0 4 0 -2 2 0 4 0", "10", "8"], ["0 -3 4 0 -2 2 0 4 0", "10", "8"], ["0 4 -3 0 -2 2 0 4 0", "10", "8"], ["0 -4 4 0 -2 2 0 4 0", "10", "8"], ["0 4 -4 0 -2 2 0 4 0", "10", "8"], ["0 4 0 2 -2 0 4 0", "10", "8"], ["0 -3 4 0 2 -2 0 4 0", "10", "8"], ["0 4 -3 0 2 -2 0 4 0", "10", "8"], ["0 -4 4 0 2 -2 0 4 0", "10", "8"], ["0 4 -4 0 2 -2 0 4 0", "10", "8"], ["0 4 0 2 0 -3 4 0", "10", "8"], ["0 -3 4 0 2 0 -3 4 0", "10", "8"], ["0 4 -3 0 2 0 -3 4 0", "10", "8"], ["0 -4 4 0 2 0 -3 4 0", "10", "8"], ["0 4 -4 0 2 0 -3 4 0", "10", "8"], ["0 4 0 -1 2 0 -3 4 0", "10", "8"], ["0 -3 4 0 -1 2 0 -3 4 0", "10", "8"], ["0 4 -3 0 -1 2 0 -3 4 0", "10", "8"], ["0 -4 4 0 -1 2 0 -3 4 0", "10", "8"], ["0 4 -4 0 -1 2 0 -3 4 0", "10", "8"], ["0 4 0 2 -1 0 -3 4 0", "10", "8"], ["0 -3 4 0 2 -1 0 -3 4 0", "10", "8"], ["0 4 -3 0 2 -1 0 -3 4 0", "10", "8"], ["0 -4 4 0 2 -1 0 -3 4 0", "10", "8"], ["0 4 -4 0 2 -1 0 -3 4 0", "10", "8"], ["0 4 0 -2 2 0 -3 4 0", "10", "8"], ["0 -3 4 0 -2 2 0 -3 4 0", "10", "8"], ["0 4 -3 0 -2 2 0 -3 4 0", "10", "8"], ["0 -4 4 0 -2 2 0 -3 4 0", "10", "8"], ["0 4 -4 0 -2 2 0 -3 4 0", "10", "8"], ["0 4 0 2 -2 0 -3 4 0", "10", "8"], ["0 -3 4 0 2 -2 0 -3 4 0", "10", "8"], ["0 4 -3 0 2 -2 0 -3 4 0", "10", "8"], ["0 -4 4 0 2 -2 0 -3 4 0", "10", "8"], ["0 4 -4 0 2 -2 0 -3 4 0", "10", "8"], ["0 4 0 2 0 4 -3 0", "10", "8"], ["0 -3 4 0 2 0 4 -3 0", "10", "8"], ["0 4 -3 0 2 0 4 -3 0", "10", "8"], ["0 -4 4 0 2 0 4 -3 0", "10", "8"], ["0 4 -4 0 2 0 4 -3 0", "10", "8"], ["0 4 0 -1 2 0 4 -3 0", "10", "8"], ["0 -3 4 0 -1 2 0 4 -3 0", "10", "8"], ["0 4 -3 0 -1 2 0 4 -3 0", "10", "8"], ["0 -4 4 0 -1 2 0 4 -3 0", "10", "8"], ["0 4 -4 0 -1 2 0 4 -3 0", "10", "8"], ["0 4 0 2 -1 0 4 -3 0", "10", "8"], ["0 -3 4 0 2 -1 0 4 -3 0", "10", "8"], ["0 4 -3 0 2 -1 0 4 -3 0", "10", "8"], ["0 -4 4 0 2 -1 0 4 -3 0", "10", "8"], ["0 4 -4 0 2 -1 0 4 -3 0", "10", "8"], ["0 4 0 -2 2 0 4 -3 0", "10", "8"], ["0 -3 4 0 -2 2 0 4 -3 0", "10", "8"], ["0 4 -3 0 -2 2 0 4 -3 0", "10", "8"], ["0 -4 4 0 -2 2 0 4 -3 0", "10", "8"], ["0 4 -4 0 -2 2 0 4 -3 0", "10", "8"], ["0 4 0 2 -2 0 4 -3 0", "10", "8"], ["0 -3 4 0 2 -2 0 4 -3 0", "10", "8"], ["0 4 -3 0 2 -2 0 4 -3 0", "10", "8"], ["0 -4 4 0 2 -2 0 4 -3 0", "10", "8"], ["0 4 -4 0 2 -2 0 4 -3 0", "10", "8"], ["0 4 0 2 0 -4 4 0", "10", "8"], ["0 -3 4 0 2 0 -4 4 0", "10", "8"], ["0 4 -3 0 2 0 -4 4 0", "10", "8"], ["0 -4 4 0 2 0 -4 4 0", "10", "8"], ["0 4 -4 0 2 0 -4 4 0", "10", "8"], ["0 4 0 -1 2 0 -4 4 0", "10", "8"], ["0 -3 4 0 -1 2 0 -4 4 0", "10", "8"], ["0 4 -3 0 -1 2 0 -4 4 0", "10", "8"], ["0 -4 4 0 -1 2 0 -4 4 0", "10", "8"], ["0 4 -4 0 -1 2 0 -4 4 0", "10", "8"], ["0 4 0 2 -1 0 -4 4 0", "10", "8"], ["0 -3 4 0 2 -1 0 -4 4 0", "10", "8"], ["0 4 -3 0 2 -1 0 -4 4 0", "10", "8"], ["0 -4 4 0 2 -1 0 -4 4 0", "10", "8"], ["0 4 -4 0 2 -1 0 -4 4 0", "10", "8"], ["0 4 0 -2 2 0 -4 4 0", "10", "8"], ["0 -3 4 0 -2 2 0 -4 4 0", "10", "8"], ["0 4 -3 0 -2 2 0 -4 4 0", "10", "8"], ["0 -4 4 0 -2 2 0 -4 4 0", "10", "8"], ["0 4 -4 0 -2 2 0 -4 4 0", "10", "8"], ["0 4 0 2 -2 0 -4 4 0", "10", "8"], ["0 -3 4 0 2 -2 0 -4 4 0", "10", "8"], ["0 4 -3 0 2 -2 0 -4 4 0", "10", "8"], ["0 -4 4 0 2 -2 0 -4 4 0", "10", "8"], ["0 4 -4 0 2 -2 0 -4 4 0", "10", "8"], ["0 4 0 2 0 4 -4 0", "10", "8"], ["0 -3 4 0 2 0 4 -4 0", "10", "8"], ["0 4 -3 0 2 0 4 -4 0", "10", "8"], ["0 -4 4 0 2 0 4 -4 0", "10", "8"], ["0 4 -4 0 2 0 4 -4 0", "10", "8"], ["0 4 0 -1 2 0 4 -4 0", "10", "8"], ["0 -3 4 0 -1 2 0 4 -4 0", "10", "8"], ["0 4 -3 0 -1 2 0 4 -4 0", "10", "8"], ["0 -4 4 0 -1 2 0 4 -4 0", "10", "8"], ["0 4 -4 0 -1 2 0 4 -4 0", "10", "8"], ["0 4 0 2 -1 0 4 -4 0", "10", "8"], ["0 -3 4 0 2 -1 0 4 -4 0", "10", "8"], ["0 4 -3 0 2 -1 0 4 -4 0", "10", "8"], ["0 -4 4 0 2 -1 0 4 -4 0", "10", "8"], ["0 4 -4 0 2 -1 0 4 -4 0", "10", "8"], ["0 4 0 -2 2 0 4 -4 0", "10", "8"], ["0 -3 4 0 -2 2 0 4 -4 0", "10", "8"], ["0 4 -3 0 -2 2 0 4 -4 0", "10", "8"], ["0 -4 4 0 -2 2 0 4 -4 0", "10", "8"], ["0 4 -4 0 -2 2 0 4 -4 0", "10", "8"], ["0 4 0 2 -2 0 4 -4 0", "10", "8"], ["0 -3 4 0 2 -2 0 4 -4 0", "10", "8"], ["0 4 -3 0 2 -2 0 4 -4 0", "10", "8"], ["0 -4 4 0 2 -2 0 4 -4 0", "10", "8"], ["0 4 -4 0 2 -2 0 4 -4 0", "10", "8"]]
  in  "16 groups":string[][](array[string])=array2000x3[6000 elements]
  out "Array 4":string[][](array[string])
  out "Slide 2":dbl(slide) scale=0.0..1.0
  out "Slide":dbl(slide) scale=0.0..2037.0
  in  "Path":path
  in  "all rows":string[][](array[string])=array2038x3[6114 elements]
  out "LCS/min (Lsample,Lknown)":dbl[][](array[numeric])
  out "Distance values (LCS)":dbl[][](array[numeric])
  out "size(s)":i32
  out "accuracy":string[][](array[string])
  out "Results":string[][](array[string])
  out "test data (K)":string[][](array[string])
  out "training data (k-1)":string[][](array[string])
  in  "K folds K":i32=10
  out "K folds data":string[][](array[string])
  out "Assigned using LCS (enhanced)":string[][](array[string])
  out "Assigned using LCS":string[][](array[string])
  in  "class labels for training data":string[](array[string])
  in  "kNN k":i32=5
  in  "training data (cluster centers)":string[](array[string])
  in  "test data (patterns in)":string[](array[string])=["0 4 0", "4 0 4", "0 4 0", "4 0 4", "0 4 0", "4 0 4", "0 4 0", "4 0 -2", "0 -2 3", "-2 3 0", "3 0 3", "0 3 0", "3 0 4", "0 4 0", "-2 0 1", "0 1 0", "1 0 -4", "0 -4 4", "-2 2 0", "2 0 -1", "0 -1 -4", "-1 -4 1", "-4 1 0", "1 0 3", "0 3 0", "-1 0 -1", "0 -1 2", "0 -1 1", "-1 1 0", "1 0 4", "0 4 0", "4 0 3", "0 3 -2", "3 -2 0", "-2 0 -2", "0 -2 3", "-2 3 -2", "3 -2 0", "-2 0 4", "0 4 0", "4 0 -2", "0 -2 2", "2 -1 0", "-1 0 4", "0 4 0", "4 0 2", "0 2 0", "2 0 -2", "0 -2 0", "1 -1 0", "-1 0 3", "0 3 0", "3 0 -4", "0 -4 4", "-4 4 -4", "4 -4 0", "2 -1 0", "-1 0 3", "0 3 -2", "3 -2 0", "-2 0 -3", "0 -3 0", "-3 0 3", "0 3 0", "3 0 -3", "0 -3 0", "0 4 0", "4 0 4", "0 4 -4", "4 -4 1", "-4 1 -1", "1 -1 0", "-1 0 -3", "0 -3 0", "-3 0 1", "0 1 -4", "1 -4 1", "-4 1 0", "1 0 4", "0 4 0", "4 0 -4", "0 -4 0", "-4 0 -4", "0 -4 4", "-4 4 -4", "4 -4 1", "0 -4 1", "-4 1 0", "1 0 -4", "0 -4 4", "0 4 0", "4 0 -2", "0 -2 2", "-2 2 -2", "2 -2 2", "-2 2 -2", "2 -2 2", "-2 2 -1", "2 -1 0", "-1 0 4", "0 4 0", "4 0 2", "0 2 0", "2 0 4", "0 4 0", "4 0 2", "0 2 -2", "2 -2 0", "-2 0 4", "1 0 -1", "0 -1 0", "-1 0 -1", "0 -1 0", "-1 0 1", "0 1 -1", "-2 2 -2", "2 -2 3", "1 0 -1", "0 -1 0", "-1 0 -1", "0 -1 2", "-1 2 0", "2 0 2", "0 2 -2", "2 -2 0", "-2 0 -4", "0 -4 0", "-2 2 0", "2 0 3", "0 3 -2", "3 -2 2", "1 -1 0", "-1 0 3", "0 4 0", "-2 0 1", "0 1 -4", "1 -4 0", "-4 0 -3", "0 -3 0", "1 0 -1", "0 -1 2", "-1 2 -1", "2 -1 1", "-1 1 -4", "-2 0 -1", "0 -1 1", "0 3 0", "3 0 3", "0 3 0", "3 0 3", "0 3 -2", "-4 0 -4", "0 -4 4", "0 4 0", "4 0 -4", "0 -4 0", "-4 0 -4", "-2 2 0", "2 0 4", "0 4 -4", "4 -4 0", "-4 0 2", "0 2 -2"]
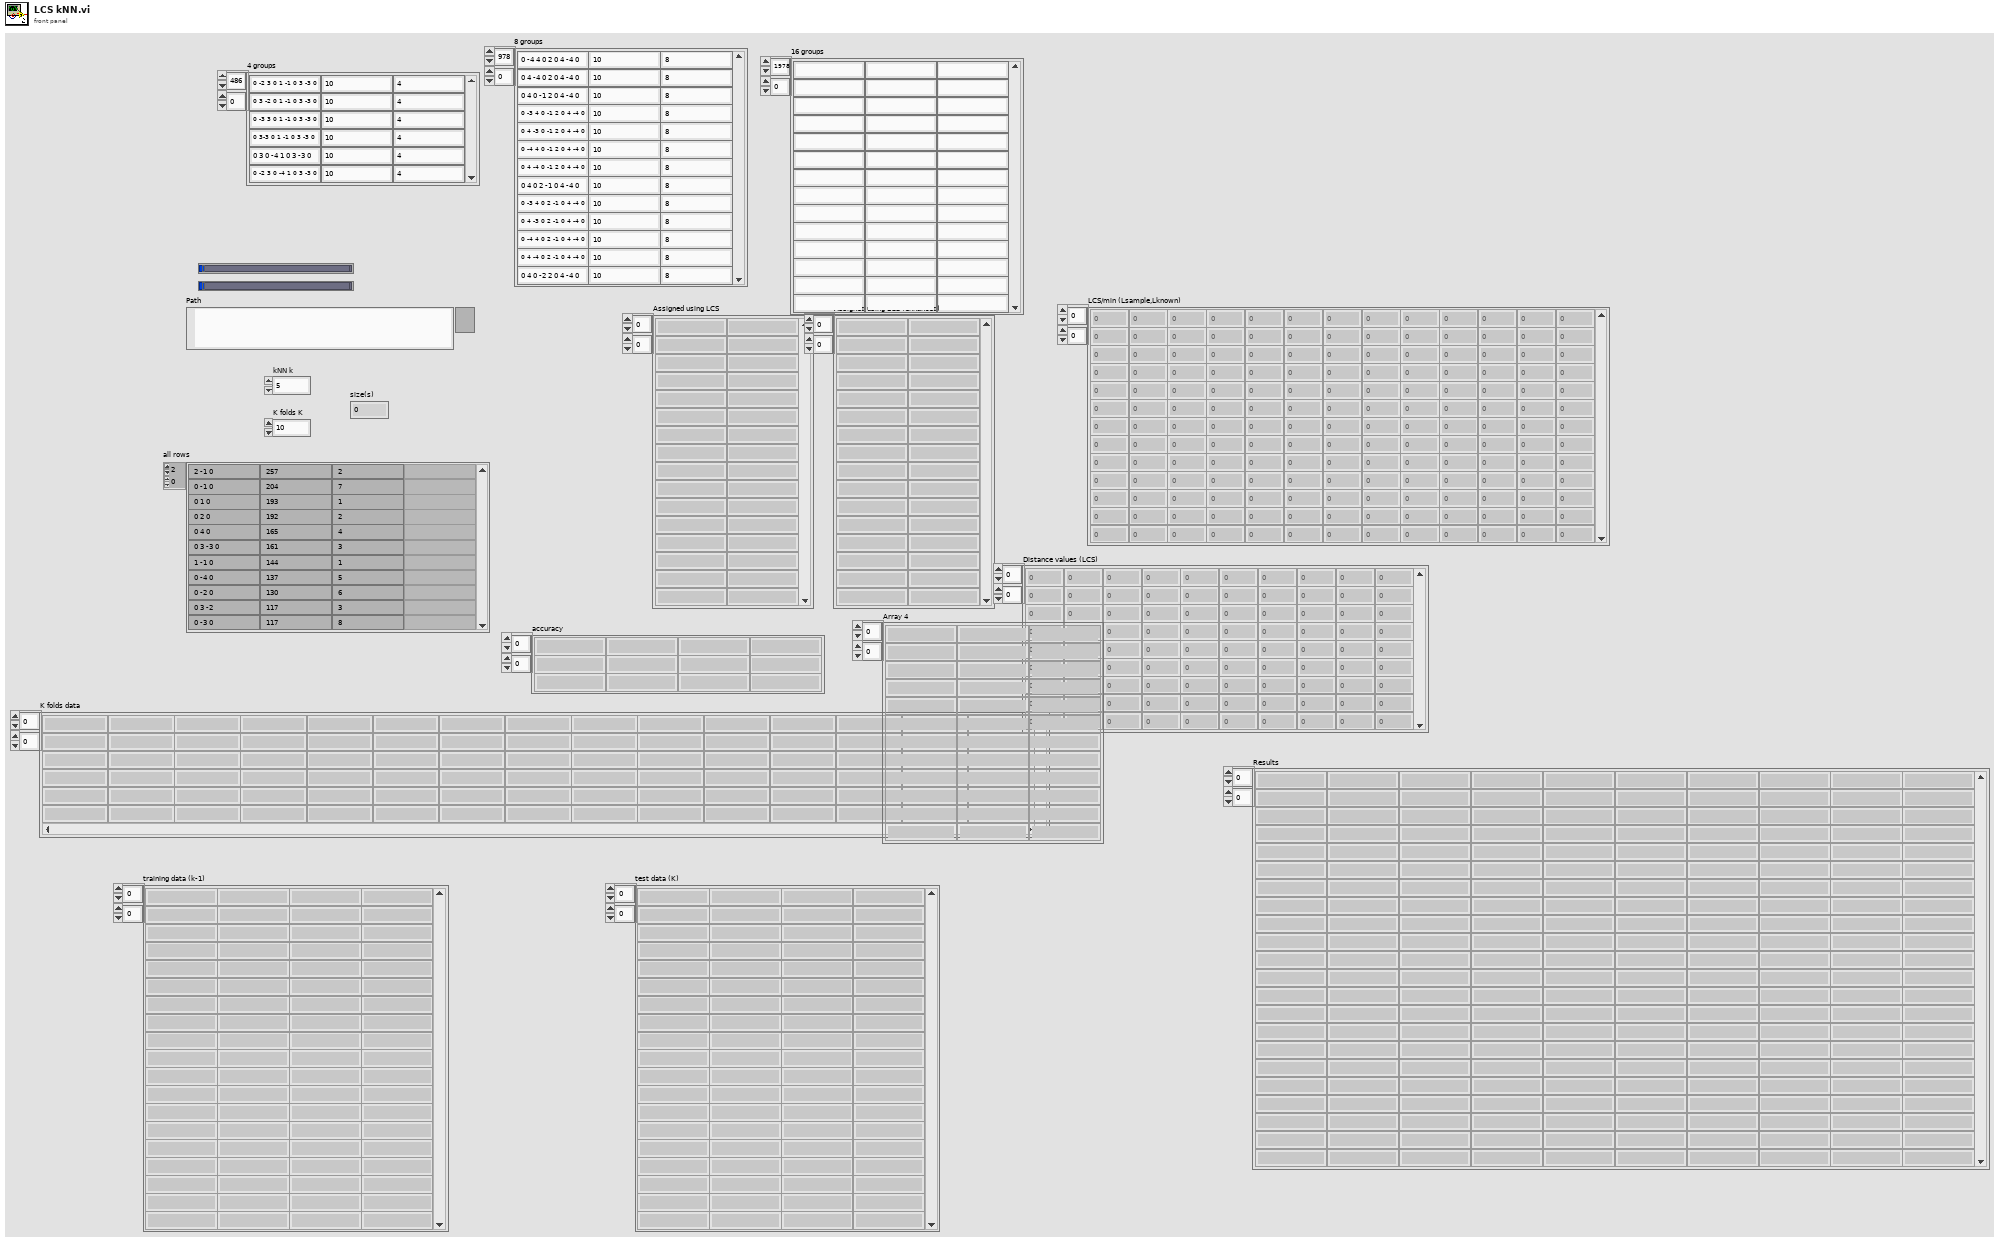
[diagram p1: front panel]
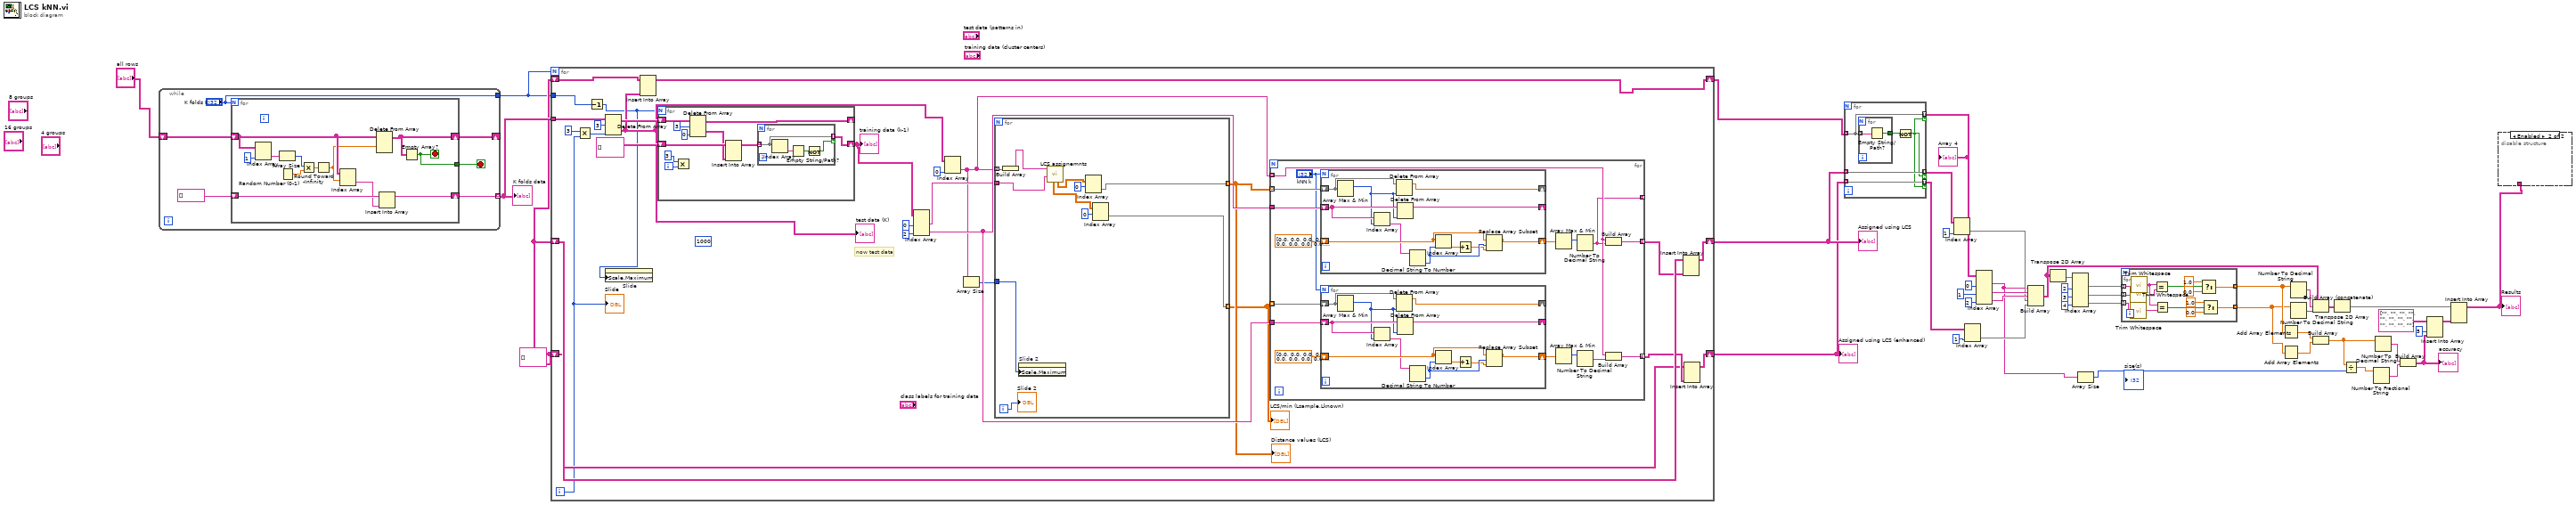
[diagram p0: block diagram]
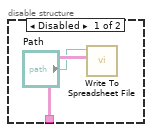
[diagram p2: hidden frame]
diagram:
  w10 = string[][] []
  n1 = while {
    shift-right: [w49] -> _
    shift-left: "all rows" -> [w50]
    tunnel: [w51] -> w46 mode=indexing
    tunnel: ["K folds K"] -> w2
    stop <- w48 stop-if-true
    n2 = for {
      N: "K folds K" -> [_]
      shift-right: [w57] -> w51
      shift-left: string[] [] ("all rows 2") -> [w64]
      shift-right: [w55] -> w49
      shift-left: w50 -> [w56]
      tunnel: [w54] -> w48
      stop <- w54 stop-if-true
      n3 = Index Array(array=w56, index (col)=1 ("disabled index (col)")) -> (element=w60:string[])  [unwired: 1 in]
      n4 = Array Size(array=w60) -> (size(s)=w61:i32)
      n5 = Random Number (0-1)() -> (number: 0 to 1=w62:dbl)
      n6 = Multiply(x=w61, y=w62) -> (x*y=w63:dbl)
      n7 = Round Toward -Infinity(1:w63) -> (0:w53:dbl)
      n8 = Index Array(array=w56, index (row)=w53) -> (element=w58:string[])  [unwired: 1 in]
      n9 = Delete From Array(array=w56, index (row)=w53) -> (array with subset deleted=w55:string[][])  [unwired: 2 in, 1 out]
      n10 = Insert Into Array(array=w64, new element=w58) -> (w57:string[])  [unwired: 1 in]
      n11 = Empty Array?(array=w55) -> (empty?=w54:bool)
    }
  }
  "K folds data" <- w46
  n12 = for {
    N: w2 -> [_]
    tunnel: w46 -> [w92]
    tunnel: w2 -> [w69]
    shift-right: [w76] -> w8
    shift-left: w10 -> [w78]
    shift-right: [w73] -> w7
    shift-left: w10 -> [w75]
    shift-right: [w70] -> w5
    shift-left: w10 -> [w71]
    i -> [w68]
    (unwired) u32 1000 ("milliseconds to wait")
    # "now test data"
    n13 = Multiply(x=3, y=w68) -> (x*y=w81:i32)
    n14 = Decrement(x=w69) -> (x-1=w65:i32)
    n15 = Delete From Array(array=w92, length=3, index (col)=w81) -> (deleted portion=w77:string[][], array with subset deleted=w80:string[][])  [unwired: 1 in]
    "test data (K)" <- w77
    n16 = property on="Slide" class="Slide (strict)"("Scale.Maximum"=w65) -> ()  [unwired: 2 in, 2 out]
    n17 = Insert Into Array(array=w78, new element=w77) -> (w76:string[][])  [unwired: 2 in]
    n18 = for {
      N: w65 -> [_]
      shift-right: [w93] -> w84
      shift-left: string[][] [] ("all rows 2") -> [w101]
      shift-right: [w96] -> _
      shift-left: w80 -> [w102]
      i -> [w98]
      n19 = Multiply(x=3, y=w98) -> ()  [unwired: 1 out]
      n20 = Delete From Array(array=w102, length=3 ("index (col)"), index (col)=0 ("disabled index (col)")) -> (deleted portion=w100:string[][], array with subset deleted=w96:string[][])  [unwired: 1 in]
      n21 = Insert Into Array(array=w101, new element=w100) -> (w94:string[][])  [unwired: 2 in]
      n22 = for {
        tunnel: w94 -> [w105] mode=indexing
        tunnel: [w105] -> w93 mode=indexing if=w106
        n23 = Index Array(array=w105) -> (element=w104:string)  [unwired: 1 in]
        n24 = Empty String/Path?(string/path=w104) -> (empty?=w103:bool)
        n25 = Not(x=w103) -> (.not. x?=w106:bool)
      }
    }
    "training data (k-1)" <- w84
    n26 = Index Array(array=w84, index (col) #1=0 ("disabled index (col)"), index (col) #2=2 ("index (col)")) -> (element #1=w87:string[], element #2=w88:string[])  [unwired: 2 in]
    n27 = Index Array(array=w77, index (col)=0 ("disabled index (col)")) -> (element=w67:string[])  [unwired: 1 in]
    n28 = Array Size(array=w67) -> (size(s)=w66:i32)
    n29 = for {
      tunnel: w67 -> [w155] mode=indexing
      tunnel: w87 -> [w150]
      tunnel: [w148] -> w86 mode=indexing
      tunnel: [w147] -> w85 mode=indexing
      tunnel: w66 -> [w153]
      i -> [w154]
      n30 = Build Array(w155) -> (w151:string[])
      n31 = property on="Slide 2" class="Slide (strict)"("Scale.Maximum"=w153) -> ()  [unwired: 2 in, 2 out]
      n32 = call "LCS assignemnts.vi"("cluster centers"=w150, "Patterns in"=w151) -> ("Distance values (LCS)"=w146:dbl[][], "LCS/LA+LB-LCS"=w145:dbl[][])  [unwired: 1 in, 7 out]
      n33 = Index Array(array=w146, index (row)=0) -> (element=w148:dbl[])  [unwired: 1 in]
      n34 = Index Array(array=w145, index (row)=0) -> (element=w147:dbl[])  [unwired: 1 in]
      "Slide 2" <- w154
    }
    "Distance values (LCS)" <- w86
    "LCS/min (Lsample,Lknown)" <- w85
    n35 = for {
      tunnel: w67 -> [w115] mode=indexing
      tunnel: w86 -> [w122] mode=indexing
      tunnel: w88 -> [w121]
      tunnel: w85 -> [w114] mode=indexing
      tunnel: w88 -> [w113]
      tunnel: [w112] -> w74 mode=indexing
      tunnel: [w111] -> w72 mode=indexing
      tunnel: [w109] -> _ mode=indexing
      n36 = for {
        N: "kNN k" -> [_]
        shift-right: [w141] -> _
        shift-left: w122 -> [w144]
        shift-right: [w140] -> _
        shift-left: w121 -> [w143]
        shift-right: [w135] -> w119
        shift-left: dbl[] [0.0, 0.0, 0.0, 0.0, 0.0, 0.0, 0.0, 0.0, 0.0, 0.0, 0.0, 0.0] -> [w136]
        n37 = Array Max & Min(array=w144) -> (max index (indices)=w142:i32)  [unwired: 3 out]
        n38 = Index Array(array=w143, index=w142) -> (element=w134:string)
        n39 = Delete From Array(array=w144, index=w142) -> (array with subset deleted=w141:dbl[])  [unwired: 1 in, 1 out]
        n40 = Delete From Array(array=w143, index=w142) -> (array with subset deleted=w140:string[])  [unwired: 1 in, 1 out]
        n41 = Decimal String To Number(string=w134) -> (number=w139:i32)  [unwired: 2 in, 1 out]
        n42 = Index Array(array=w136, index=w139) -> (element=w137:dbl)
        n43 = Increment(x=w137) -> (x+1=w138:dbl)
        n44 = Replace Array Subset(array=w136, new element=w138, index=w139) -> (w135:dbl[])
      }
      n45 = for {
        N: "kNN k" -> [_]
        shift-right: [w130] -> _
        shift-left: w114 -> [w133]
        shift-right: [w129] -> _
        shift-left: w113 -> [w132]
        shift-right: [w124] -> w117
        shift-left: dbl[] [0.0, 0.0, 0.0, 0.0, 0.0, 0.0, 0.0, 0.0, 0.0, 0.0, 0.0, 0.0] -> [w125]
        n46 = Array Max & Min(array=w133) -> (max index (indices)=w131:i32)  [unwired: 3 out]
        n47 = Index Array(array=w132, index=w131) -> (element=w123:string)
        n48 = Delete From Array(array=w133, index=w131) -> (array with subset deleted=w130:dbl[])  [unwired: 1 in, 1 out]
        n49 = Delete From Array(array=w132, index=w131) -> (array with subset deleted=w129:string[])  [unwired: 1 in, 1 out]
        n50 = Decimal String To Number(string=w123) -> (number=w128:i32)  [unwired: 2 in, 1 out]
        n51 = Index Array(array=w125, index=w128) -> (element=w126:dbl)
        n52 = Increment(x=w126) -> (x+1=w127:dbl)
        n53 = Replace Array Subset(array=w125, new element=w127, index=w128) -> (w124:dbl[])
      }
      n54 = Array Max & Min(array=w119) -> (max index (indices)=w120:i32)  [unwired: 3 out]
      n55 = Array Max & Min(array=w117) -> (max index (indices)=w116:i32)  [unwired: 3 out]
      n56 = Number To Decimal String(number=w120) -> (decimal integer string=w109:string)  [unwired: 1 in]
      n57 = Number To Decimal String(number=w116) -> (decimal integer string=w118:string)  [unwired: 1 in]
      n58 = Build Array(w115, w109) -> (w112:string[])
      n59 = Build Array(w115, w118) -> (w111:string[])
    }
    n60 = Insert Into Array(array=w75, new element=w74) -> (w73:string[][])  [unwired: 2 in]
    n61 = Insert Into Array(array=w71, new element=w72) -> (w70:string[][])  [unwired: 2 in]
    "Slide" <- w68
  }
  "Assigned using LCS" <- w7
  "Assigned using LCS (enhanced)" <- w5
  n62 = for {
    tunnel: w8 -> [w159] mode=indexing
    tunnel: [w159] -> w6 mode=indexing if=w156
    tunnel: w7 -> [w158] mode=indexing
    tunnel: [w158] -> w3 mode=indexing if=w156
    tunnel: [w157] -> w4 mode=indexing if=w156
    tunnel: w5 -> [w157] mode=indexing
    n63 = for {
      tunnel: w159 -> [w162] mode=indexing
      tunnel: [w161] -> w160
      n64 = Empty String/Path?(string/path=w162) -> (empty?=w161:bool)
    }
    n65 = Not(x=w160) -> (.not. x?=w156:bool)
  }
  "Array 4" <- w6
  n66 = Index Array(array=w3, index (col)=1 ("disabled index (col)")) -> (element=w16:string[])  [unwired: 1 in]
  n67 = Index Array(array=w4, index (col)=1 ("disabled index (col)")) -> (element=w14:string[])  [unwired: 1 in]
  n68 = Index Array(array=w6, index (col) #1=0 ("disabled index (col)"), index (col) #2=1 ("index (col)"), index (col) #3=2 ("index (col)")) -> (element #1=w12:string[], element #2=w19:string[], element #3=w18:string[])  [unwired: 3 in]
  n69 = Build Array(w12, w19, w18, w16, w14) -> (w13:string[][])
  n70 = Transpose 2D Array(2D array=w13) -> (transposed array=w37:string[][])
  n71 = Index Array(array=w37, index (col) #1=2 ("disabled index (col)"), index (col) #2=3 ("index (col)"), index (col) #3=4 ("index (col)")) -> (element #1=w40:string[], element #2=w39:string[], element #3=w38:string[])  [unwired: 3 in]
  n72 = Array Size(array=w12) -> (size(s)=w11:i32)
  "size(s)" <- w11
  n73 = for {
    tunnel: w40 -> [w168] mode=indexing
    tunnel: w39 -> [w167] mode=indexing
    tunnel: w38 -> [w166] mode=indexing
    tunnel: [w170] -> w22 mode=indexing
    tunnel: [w169] -> w21 mode=indexing
    n74 = call <vilib>:"Trim Whitespace.vi"("string"=w167) -> ("trimmed string"=w165:string)  [unwired: 1 in]
    n75 = call <vilib>:"Trim Whitespace.vi"("string"=w166) -> ("trimmed string"=w164:string)  [unwired: 1 in]
    n76 = call <vilib>:"Trim Whitespace.vi"("string"=w168) -> ("trimmed string"=w163:string)  [unwired: 1 in]
    n77 = Equal?(x=w163, y=w165) -> (x = y?=w176:bool)
    n78 = Equal?(x=w163, y=w164) -> (x = y?=w171:bool)
    n79 = Select(t=1.0, s=w176, f=0.0) -> (s? t:f=w170:dbl)
    n80 = Select(t=1.0, s=w171, f=0.0) -> (s? t:f=w169:dbl)
  }
  n81 = Add Array Elements(numeric array=w22) -> (sum=w23:dbl)
  n82 = Add Array Elements(numeric array=w21) -> (sum=w24:dbl)
  n83 = Number To Decimal String(number=w22) -> (decimal integer string=w36:string[])  [unwired: 1 in]
  n84 = Number To Decimal String(number=w21) -> (decimal integer string=w35:string[])  [unwired: 1 in]
  n85 = Build Array (concatenate)(w13, w36, w35) -> (w34:string[][])
  n86 = Build Array(w23, w24) -> (w25:dbl[])
  n87 = Transpose 2D Array(2D array=w34) -> (transposed array=w20:string[][])
  n88 = Divide(x=w25, y=w11) -> (x/y=w26:dbl[])
  n89 = Number To Fractional String(number=w26) -> (F-format string=w28:string[])  [unwired: 3 in]
  n90 = Number To Decimal String(number=w25) -> (decimal integer string=w27:string[])  [unwired: 1 in]
  n91 = Build Array(w27, w28) -> (w32:string[][])
  "accuracy" <- w32
  n92 = Insert Into Array(array=string[][] [["", "", "", "", "", ""], ["", "", "", "", "", ""]] ("appended array 3"), index (col)=5 ("disabled index (col)"), new element=w32) -> (w31:string[][])  [unwired: 1 in]
  n93 = Insert Into Array(array=w20, new element=w31) -> (w9:string[][])  [unwired: 2 in]
  "Results" <- w9
  n94 = disable-structure shown="Enabled" {
    disable-tunnel: w9 -> [w178 _]
    frame Disabled {
      n95 = call-poly <vilib>:"Write To Spreadsheet File.vi"("2D data"=w178, "file path (dialog if empty)"="Path") -> ()  [unwired: 6 in, 1 out]
    }
    frame Enabled {
    }
  }
